vi "Create control.vi"() -> ()   [LabVIEW 2012]
uses:
  Typedefs/TypeDef_Action.ctl
  _Control Generator/BX.Orientation__LCR _Modified.ctl
  Controls/_ui_tools_font.ctl
  Control.lvclass
  <vilib>/Utility/miscctls.llb/LVPointTypeDef.ctl
  <vilib>/Palette API/Palette Menu/Public Type Define/Palette type.ctl
  <vilib>/Palette API/Palette Menu/Public Type Define/Item.ctl
  <userlib>/_OpenG.lib/array/array.llb/Conditional Auto-Indexing Tunnel (String)__ogtk.vi
  <userlib>/_OpenG.lib/file/file.llb/File Exists - Scalar__ogtk.vi
  <userlib>/_OpenG.lib/file/file.llb/Strip Path - Traditional__ogtk.vi
  <userlib>/_OpenG.lib/file/file.llb/Strip Path Extension - String__ogtk.vi
  <userlib>/_OpenG.lib/string/string.llb/To Proper Case (String)__ogtk.vi
  <vilib>/Utility/config.llb/Read Key (String).vi
  <vilib>/Utility/config.llb/Write Key (String).vi
  <vilib>/Utility/config.llb/Read Key (Boolean).vi
  <userlib>/_OpenG.lib/file/file.llb/Build Path - Traditional__ogtk.vi
  <vilib>/Utility/config.llb/NI_LVConfig.lvlib
  <vilib>/Palette API/Palette Menu/Palette Menu.lvlib
panel:
  in  "End program afterwards":bool
  in  "Save for version":u16(ring) items=["9.0", "8.6", "8.5", "8.2", "8.0"]
  in  "Save *.ctl to disk":bool
  in  "Zoom Min":bool
  in  "Zoom Max":bool
  in  "Scale Icon":dbl(slide)=1.0 min=0.5 max=2.0 scale=0.5..2.0 scale format="%.2g"
  in  "Text Color":u32(colorbox)
  in  "Palette":path=path "_LavaCR/CustomControls" caption="<user.lib>\\"
  in  "Front Panels":u16(ring)
  in  "Drop on Front Panel":bool
  in  "Font":T1={"Font Name:"="Tahoma", "Size"=13, "Strikeout?"=FALSE, "Italic?"=FALSE, "Underline?"=FALSE, "Outline?"=FALSE, "Shadow?"=FALSE, "Bold?"=TRUE}
  in  "Add a copy to UI Tools Palette":bool
  in  "Projects":u16(ring)
  in  "Add to Project":bool
  in  "Button Style":u16(ring) items=["GlassWeb", "Mac", "Mandelbrot", "OfficeXP", "Outlook", "Round", "System", "System_test", "Vista1", "Vista_medium", "Vista_small"]
  in  "Cancel":bool
  in  "Create":bool
  in  "Orientations":T2=14
  in  "Action":T3=4 items=["Switch when pressed", "Switch when released", "Switch until release", "Latch when pressed", "Latch when released", "Latch until released"]
  in  "Control Text":string
  in  "Icon source":path caption="Icon source (single PNG file or source directory for batch processing)"
  out "Controls preview":picture
  # "BATCH PROCESSING NOT IMPLEMENTED YET\nWITH THIS UTILITY VI."
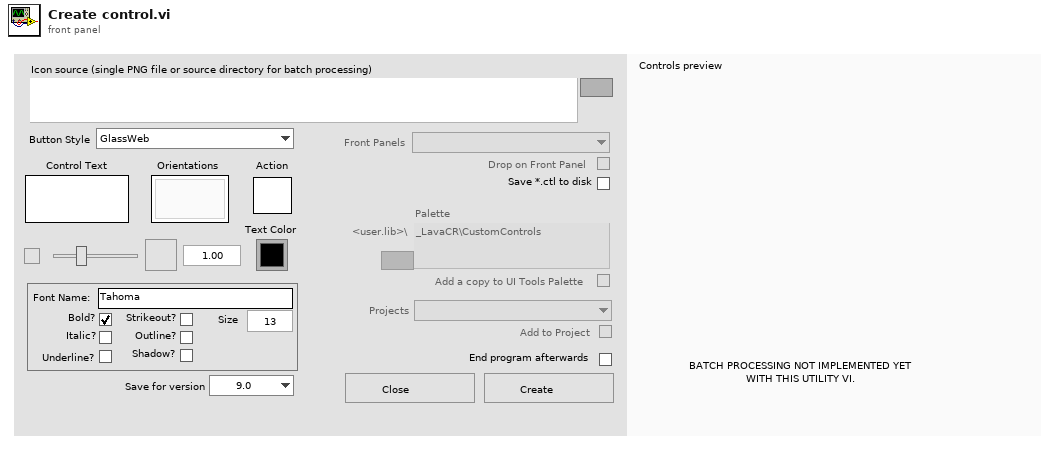
[diagram p1: front panel]
types:
  T1 = typedef "Control.lvclass/_ui_tools_font.ctl" = cluster{"Font Name:":string, "Size":i16, "Strikeout?":bool, "Italic?":bool, "Underline?":bool, "Outline?":bool, "Shadow?":bool, "Bold?":bool}
  T2 = typedef "BX.Orientation__LCR _Modified.ctl" = u8
  T3 = typedef "Control.lvclass/TypeDef_Action.ctl" = u16
  T4 = cluster{"Action":refnum<user-event>, "Orientations":refnum<user-event>, "Icon (*.png)":refnum<user-event>, "Font":refnum<user-event>, "Control Text":refnum<user-event>, "Style":refnum<user-event>, "Text Color":refnum<user-event>, "Scale Icon":refnum<user-event>}
  T5 = enum32{"invalid app kind", "Development System", "Run Time System", "Student Edition", "Embedded LabVIEW", "Evaluation", "Custom"}
  T6 = enum32{"Invalid", "Standard", "Closed", "Hidden", "Minimized", "Maximized"}
  T7 = enum32{"Bad", "Idle", "Run top level", "Running"}
  T8 = typedef "LVPointTypeDef.ctl" = cluster{"Horizontal":i16, "Vertical":i16}
  T9 = typedef "Palette Menu.lvlib/Item.ctl" = cluster{"item path":path, "library path (.lvlib)":path, "use default lvlib palette":bool, "short name":string, "place VI contents":bool, "hide synchronized item":bool, "reserve spot for synch item":bool, "configure when placing VI contents":bool}
  T10 = cluster{"Core":cluster{"Current VI Reference":refnum<vi>, "Close Panel on Exit?":bool, "NI.LV.Dialog namespace":bool, "Menu Launch:App":refnum<vi>, "Local App":refnum<vi>}, "Control":refnum<class "Control.lvclass">, "Errors":cluster{"code":i32, "Short":string, "Long":string, "Critical":bool}[], "user events":cluster{"Action":refnum<user-event>, "Orientations":refnum<user-event>, "Icon (*.png)":refnum<user-event>, "Font":refnum<user-event>, "Control Text":refnum<user-event>, "Style":refnum<user-event>, "Text Color":refnum<user-event>, "Scale Icon":refnum<user-event>}, "last state":cluster{"Action":T3, "Orientations":T2, "Icon png":path, "Control Text":string, "Style":u16, "Text Color":u32, "Scale":dbl, "Close afterwards":bool}, "config":cluster{"fade":u32, "droplabel":bool}, "file in tmp dir":path, "Source":cluster{"Icon source":path}}
  T11 = cluster{"code":i32, "Short":string, "Long":string, "Critical":bool}[]
  T12 = cluster{"Action":T3, "Orientations":T2, "Icon png":path, "Control Text":string, "Style":u16, "Text Color":u32, "Scale":dbl, "Close afterwards":bool}
  T13 = cluster{"Current VI Reference":refnum<vi>, "Close Panel on Exit?":bool, "NI.LV.Dialog namespace":bool, "Menu Launch:App":refnum<vi>, "Local App":refnum<vi>}
  T14 = typedef "NI_LVConfig.lvlib/Config Data RefNum.ctl" = refnum<k1>
  T15 = typedef "imagedata.ctl" = cluster{"image type":i32, "image depth":i32, "image":u8[], "mask":u8[], "colors":u32[], "Rectangle":cluster{"left":i16, "top":i16, "right":i16, "bottom":i16}}
  T16 = cluster{"left":i16, "top":i16, "right":i16, "bottom":i16}
  T17 = cluster{"code":i32, "Short":string, "Long":string, "Critical":bool}
  T18 = typedef "Palette Menu.lvlib/Palette type.ctl" = i32
  T19 = typedef "Palette Menu.lvlib/Palette Data.ctl" = cluster{"display name":string, "view format":T20, "palette width":i16, "items":T21, "256 color icon":picture, "B&W color icon":picture, "help information":T22, "palette description":string, "synchronize information":T23}
  T20 = typedef "Palette Menu.lvlib/View Format.ctl" = u16
  T21 = typedef "Palette Menu.lvlib/Items.ctl" = T9[]
  T22 = typedef "Palette Menu.lvlib/Help Info.ctl" = cluster{"help tag":string, "help file path ":path}
  T23 = typedef "Palette Menu.lvlib/Synchronize Info.ctl" = cluster{"synchronize with directory":bool, "synchronize directory path":path}
  T24 = typedef "Control.lvclass/BX.Orientation__LCR _Modified.ctl" = u8
  T25 = typedef "Control.lvclass/TypeDef_Styles.ctl" = u16
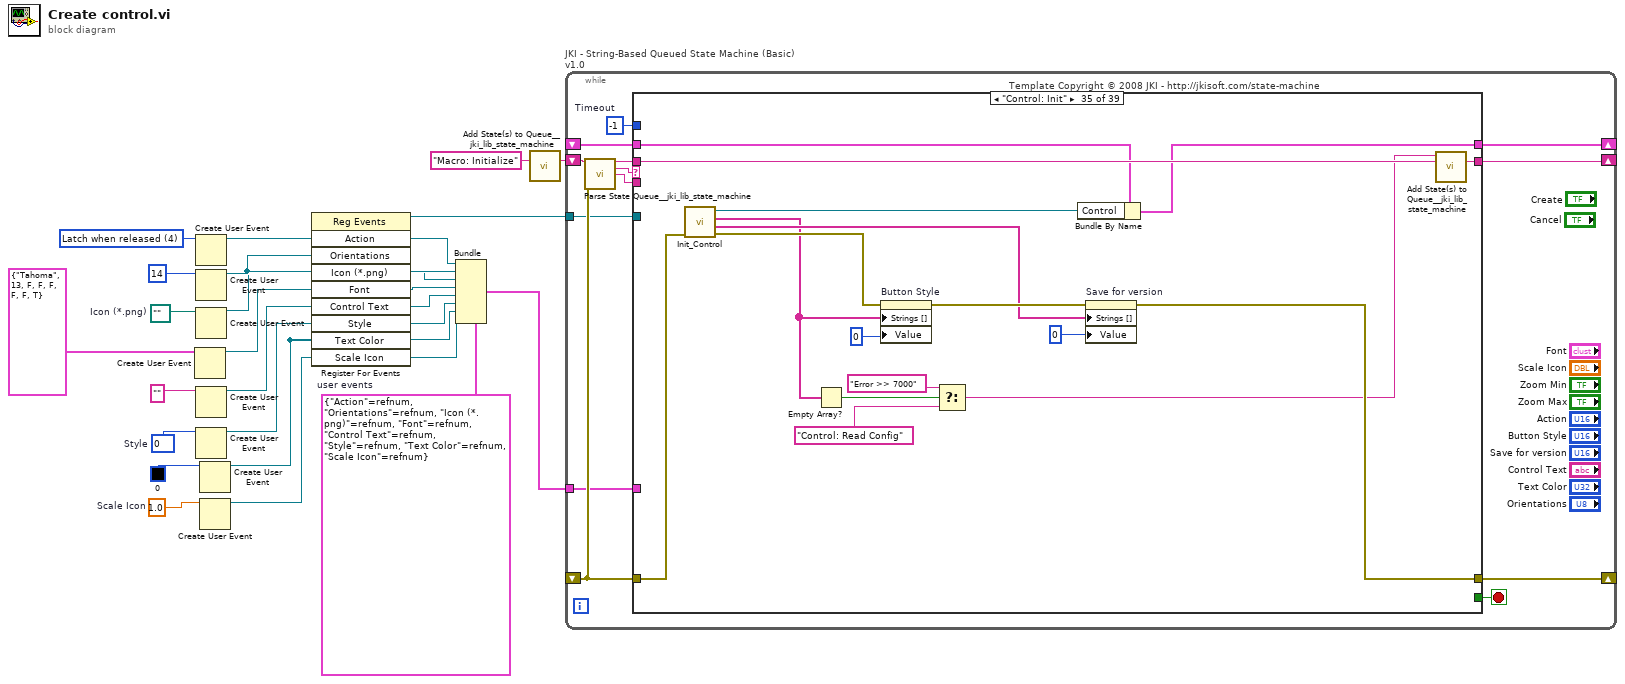
[diagram p0: block diagram]
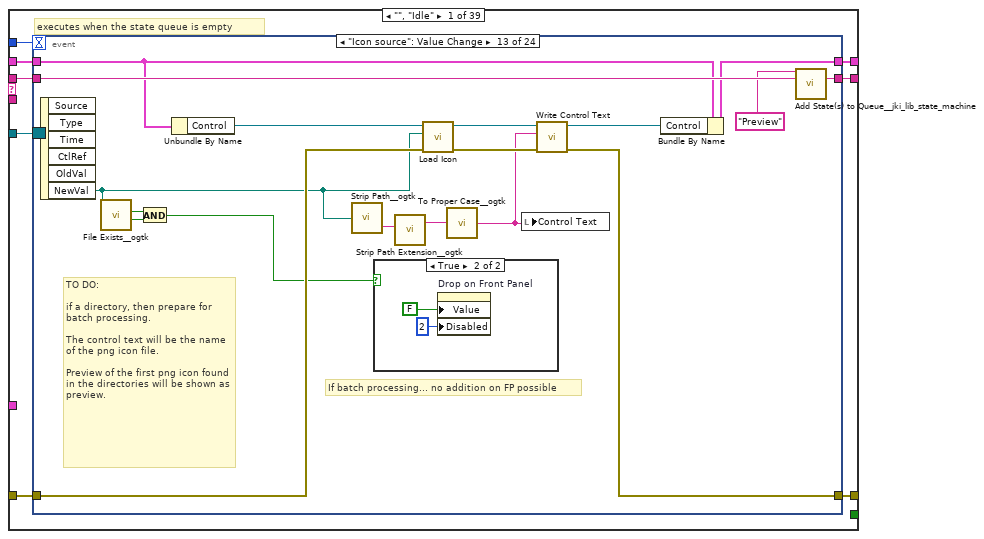
[diagram p2: hidden frame]
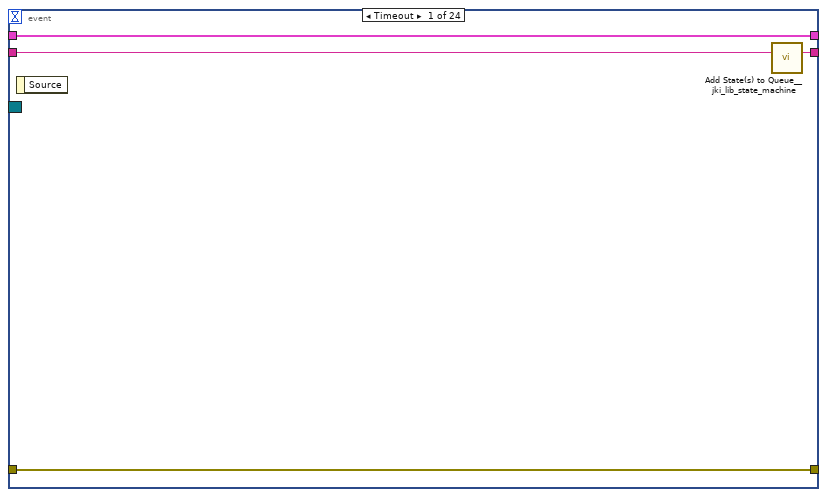
[diagram p3: hidden frame]
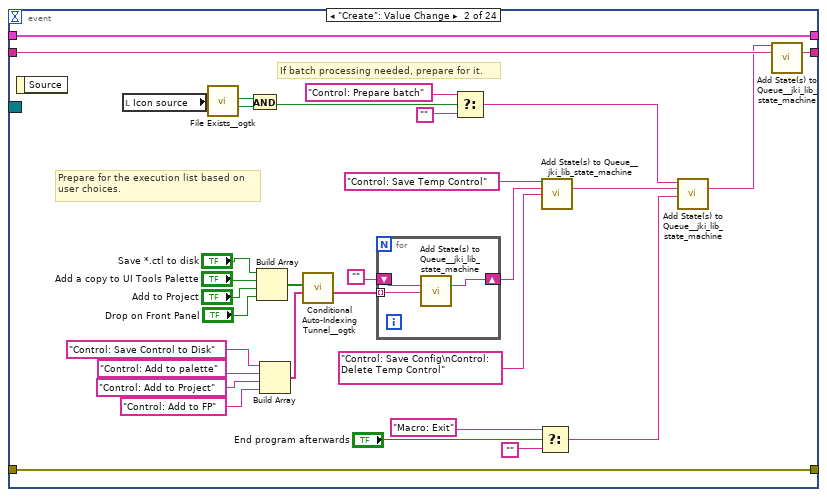
[diagram p4: hidden frame]
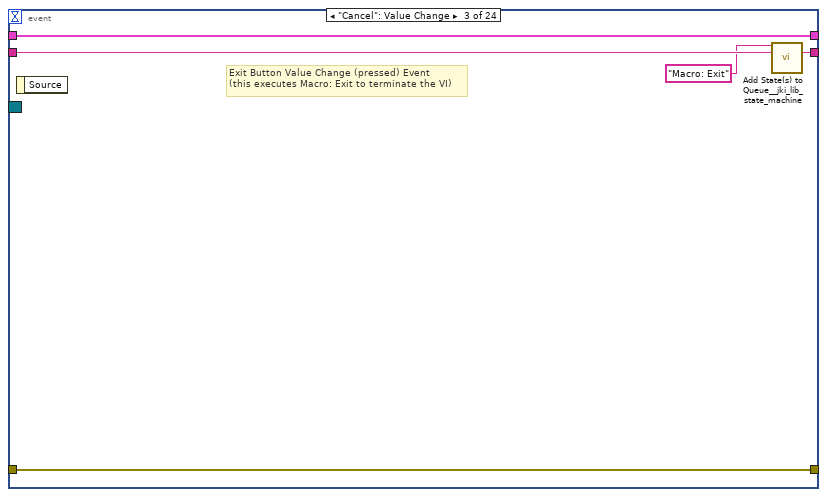
[diagram p5: hidden frame]
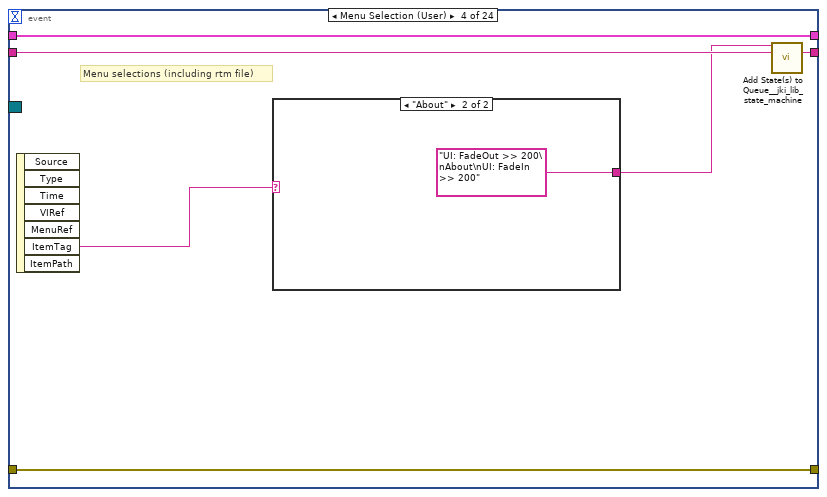
[diagram p6: hidden frame]
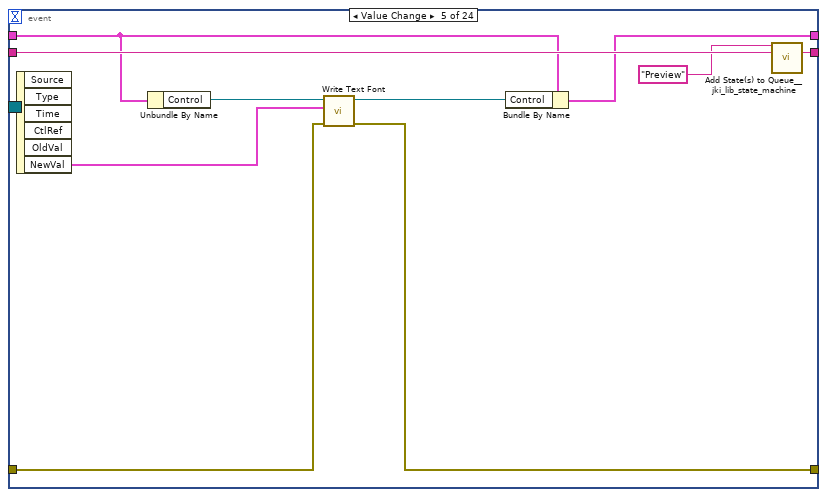
[diagram p8: hidden frame]
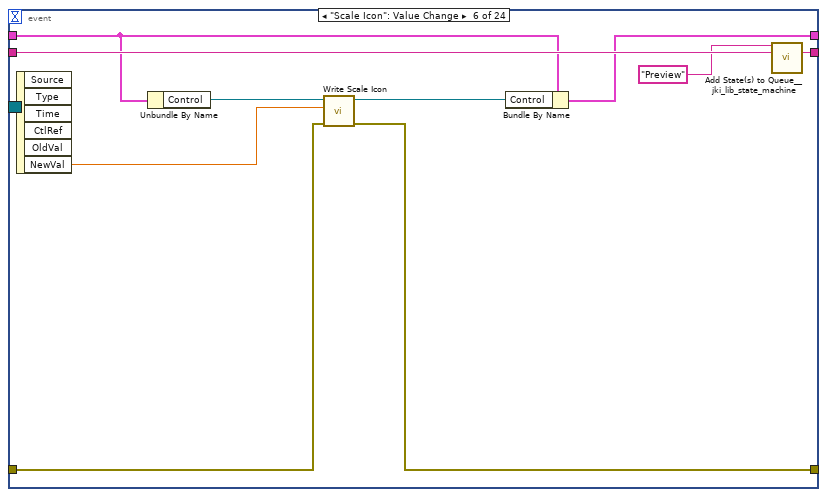
[diagram p9: hidden frame]
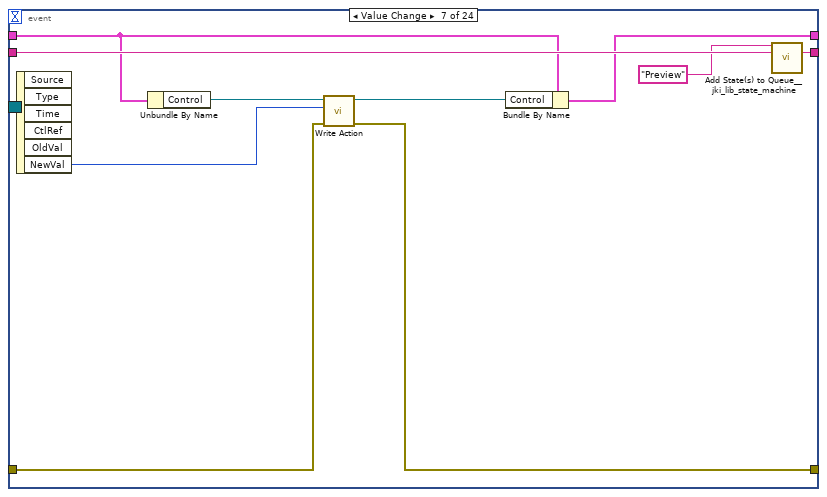
[diagram p10: hidden frame]
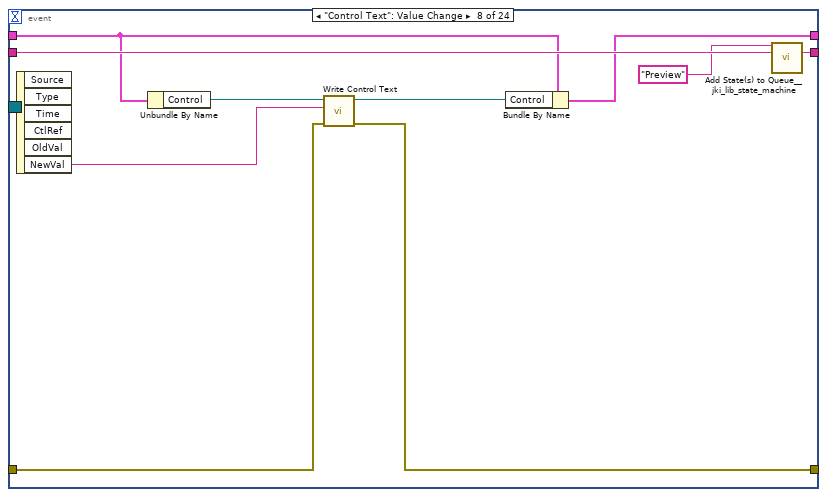
[diagram p11: hidden frame]
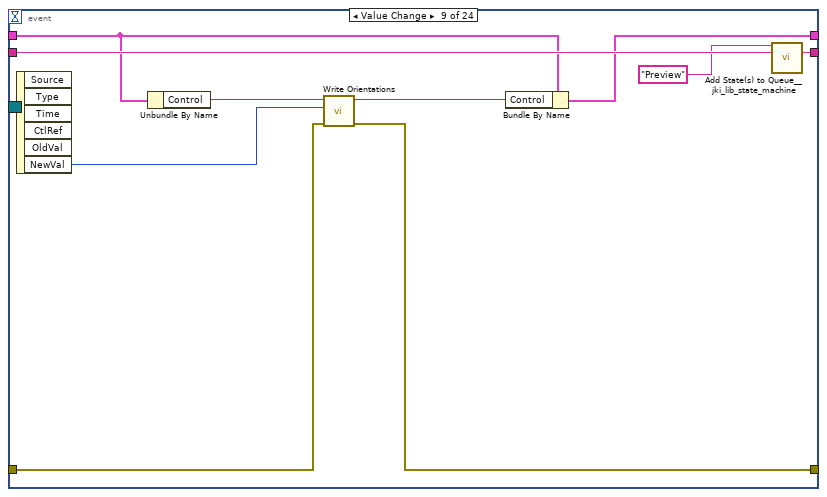
[diagram p12: hidden frame]
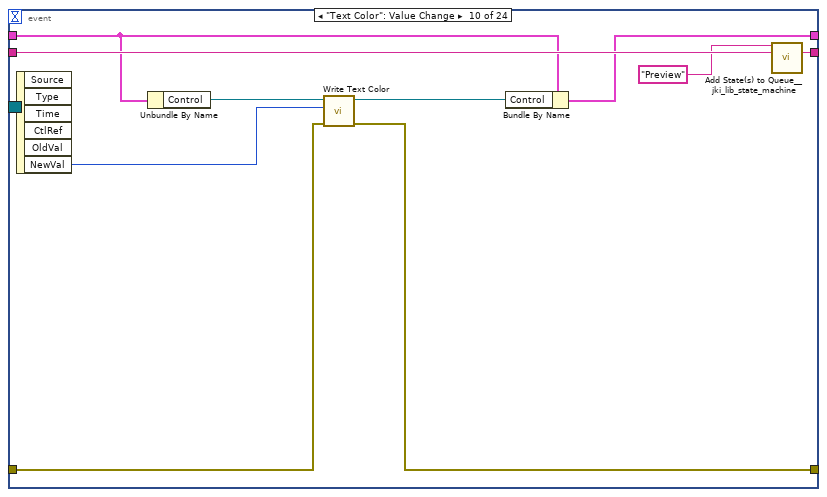
[diagram p13: hidden frame]
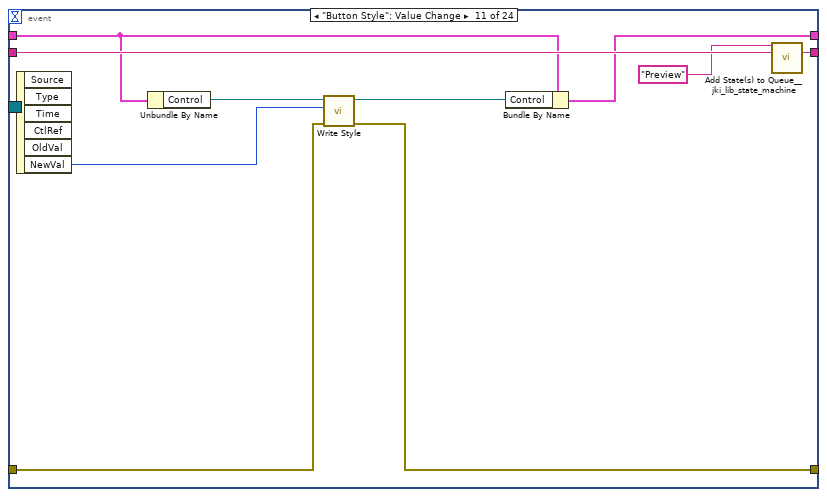
[diagram p14: hidden frame]
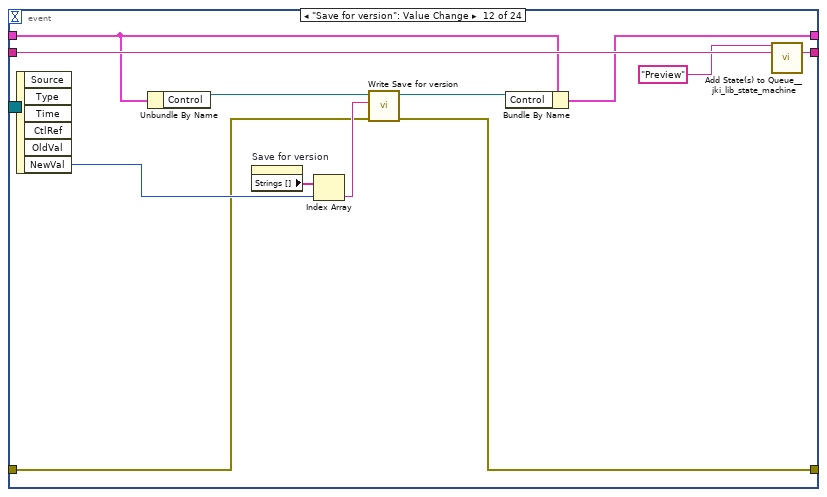
[diagram p15: hidden frame]
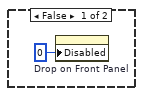
[diagram p16: hidden frame]
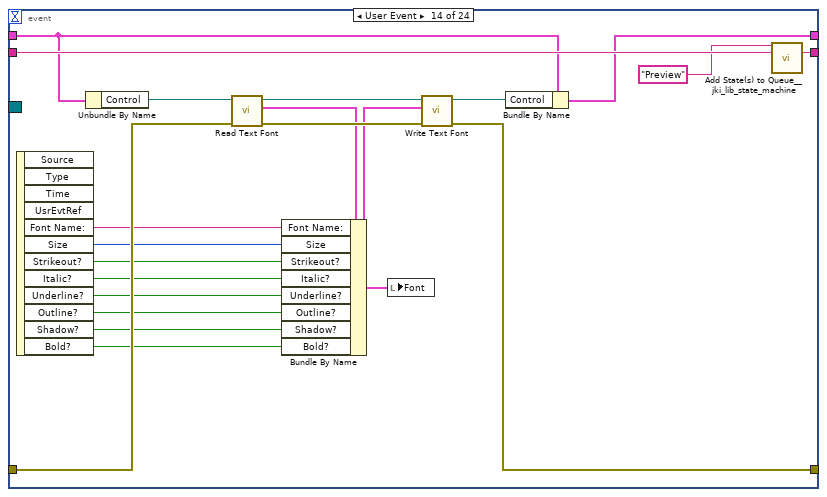
[diagram p17: hidden frame]
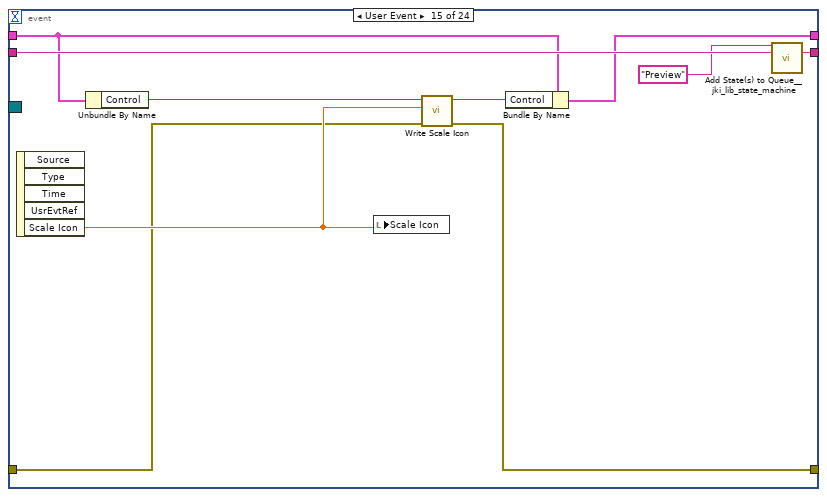
[diagram p18: hidden frame]
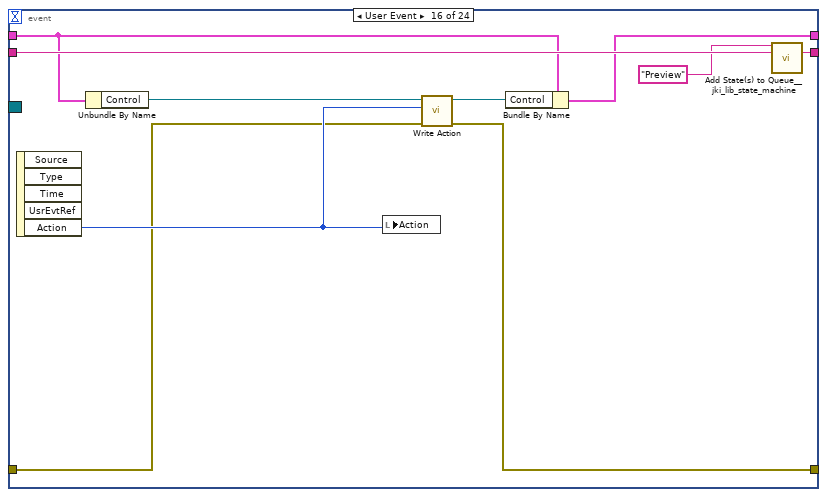
[diagram p19: hidden frame]
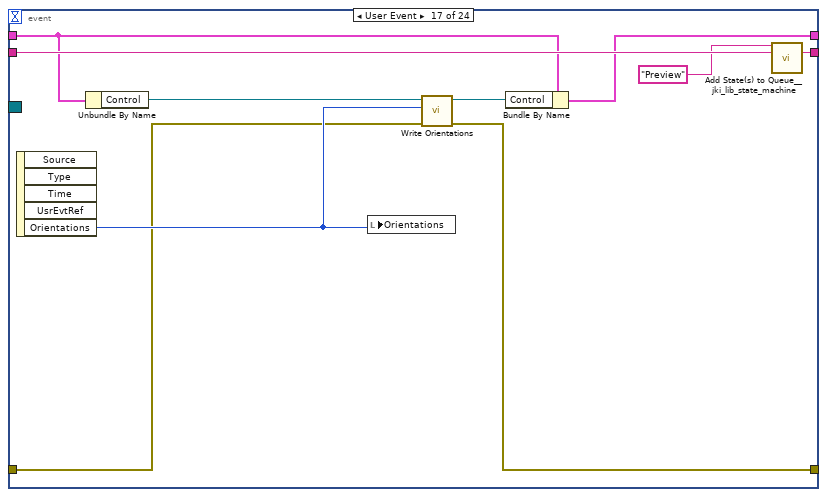
[diagram p20: hidden frame]
diagram:
  w2 = T4 {"Action"=refnum, "Orientations"=refnum, "Icon (*.png)"=refnum, "Font"=refnum, "Control Text"=refnum, "Style"=refnum, "Text Color"=refnum, "Scale Icon"=refnum}  # user events
  w7 = 1.0  # Scale Icon
  w11 = u16 0 items=[""]  # Style
  w17 = path ""  # Icon (*.png)
  w21 = T3 4 items=["Switch when pressed", "Switch when released", "Switch until release", "Latch when pressed", "Latch when released", "Latch until released"] ("Action")
  n1 = Create User Event(user event datatype=T1 {"Font Name:"="Tahoma", "Size"=13, "Strikeout?"=FALSE, "Italic?"=FALSE, "Underline?"=FALSE, "Outline?"=FALSE, "Shadow?"=FALSE, "Bold?"=TRUE} ("Font")) -> (user event=w14:refnum<user-event>)  [unwired: 1 in, 1 out]
  n2 = Create User Event(user event datatype=w21) -> (user event=w20:refnum<user-event>)  [unwired: 1 in, 1 out]
  n3 = Create User Event(user event datatype=T2 14 ("Orientations")) -> (user event=w19:refnum<user-event>)  [unwired: 1 in, 1 out]
  n4 = Create User Event(user event datatype=w17) -> (user event=w16:refnum<user-event>)  [unwired: 1 in, 1 out]
  n5 = Create User Event(user event datatype="" ("Control Text")) -> (user event=w12:refnum<user-event>)  [unwired: 1 in, 1 out]
  n6 = Create User Event(user event datatype=w11) -> (user event=w10:refnum<user-event>)  [unwired: 1 in, 1 out]
  n7 = Create User Event(user event datatype=u32 0 ("Text Color")) -> (user event=w8:refnum<user-event>)  [unwired: 1 in, 1 out]
  n8 = Create User Event(user event datatype=w7) -> (user event=w6:refnum<user-event>)  [unwired: 1 in, 1 out]
  n9 = register-events(w20, w19, w16, w14, w12, w10, w8, w6) -> (reference out=w1:refnum<event-registration>)  [unwired: 2 in, 1 out]
  n10 = Bundle(cluster=w2, "Action"=w20, "Orientations"=w19, "Icon (*.png)"=w16, "Font"=w14, "Control Text"=w12, "Style"=w10, "Text Color"=w8, "Scale Icon"=w6) -> (w3:T4)
  n11 = call <vilib>:"Add State(s) to Queue__jki_lib_state_machine.vi"("State(s) in (\"\")"="Macro: Initialize") -> ("States Out"=w5:string)  [unwired: 14 in]
  n12 = while "JKI - String-Based Queued State Machine (Basic) v1.0" {
    shift-right: [w27] -> _
    shift-left: _ -> [w26]
    shift-right: [w30] -> _
    shift-left: _ -> [w24]
    shift-right: [w29] -> _
    shift-left: w5 -> [w31]
    tunnel: w3 -> [w23]
    tunnel: w1 -> [w22]
    stop <- w28 stop-if-true
    w25 = -1  # Timeout
    # "Template Copyright © 2008 JKI - http://jkisoft.com/state-machine"
    n13 = call <vilib>:"Parse State Queue__jki_lib_state_machine.vi"("State Queue"=w31, "Error In (no error)"=w24) -> ("Remaining States"=w33:string, "Current State"=w34:string, "Arguments"=w32:string)  [unwired: 11 in]
    n14 = case shown="\"Control: Init\"" w34 {
      selector: w34 -> [_ _ w326 _ _ _ _ _ _ _ _ _ _ _ _ _ _ _ _ _ _ _ _ _ _ _ _ _ _ _ _ _ _ _ _ _ _ _ _]
      tunnel: w33 -> [w42 w325 w330 w340 w358 w368 w393 w403 w407 w419 w441 w454 w465 w492 w506 w513 w520 w526 w537 w576 w597 w620 w625 w636 w640 w661 w690 w730 w738 w761 w809 w841 w884 w904 w921 w933 w985 w1022 w1054]
      tunnel: w32 -> [_ _ _ _ _ _ w391 _ _ _ _ _ _ _ w502 _ _ w521 w531 _ _ _ _ _ _ _ _ _ _ _ _ _ _ _ _ _ _ _ _]
      tunnel: w26 -> [w40 w322 w328 w337 w349 w365 w390 w401 w404 _ w437 w451 w457 w477 w504 w511 w518 w524 w533 w561 w584 w617 w622 w628 w637 w645 w675 w727 w735 w759 w790 w839 w843 w901 w919 w934 w983 w1029 w1041]
      tunnel: [w39 w323 w332 w338 w355 errorcluster {"status"=FALSE, "code"=0, "source"=""} ("error out") w387 w400 w405 w416 w426 w452 w455 w480 w497 w508 w515 w522 w534 w574 w595 w618 w623 w626 w638 w659 w688 w728 w736 w742 w798 w831 w856 w902 w911 w939 w987 w1009 w1035] -> w30
      tunnel: w24 -> [w38 w323 w331 w338 w355 w360 _ w400 w405 w416 w438 w452 w455 w481 w498 w509 w516 w523 w535 w574 w595 w618 w623 w626 w638 w659 w688 w728 w736 w741 w797 w832 w861 w902 w912 w940 w988 w1008 w1036]
      tunnel: [w41 w324 w329 w339 w357 w367 w392 w402 w406 w418 w440 w453 w464 w491 w505 w512 w519 w525 w536 w575 w596 w619 w624 w635 w639 w660 w689 w729 w737 w760 w808 w840 w883 w903 w920 w937 w986 w1020 w1053] -> w29
      tunnel: [_ _ _ _ _ _ _ TRUE _ _ _ _ _ _ _ _ _ _ _ _ _ _ _ _ _ _ _ _ _ _ _ _ _ _ _ _ _ _ _] -> w28
      tunnel: [w37 w322 w328 w337 w356 w365 w390 w401 w404 w417 w437 w451 w457 w476 w504 w511 w518 w524 w533 w561 w584 w617 w622 w628 w637 w644 w674 w726 w734 w758 w807 w838 w882 w900 w918 w930 w984 w1029 w1040] -> w27
      tunnel: w25 -> [w36 _ _ _ _ _ _ _ _ _ _ _ _ _ _ _ _ _ _ _ _ _ _ _ _ _ _ _ _ _ _ _ _ _ _ _ _ _ _]
      tunnel: w23 -> [_ _ _ _ _ _ _ _ _ w412 _ _ _ _ _ _ _ _ _ _ _ _ _ _ _ _ _ _ _ _ _ _ _ _ _ _ _ _ _]
      tunnel: w22 -> [w35 _ _ _ _ _ _ _ _ _ w436 _ _ _ _ _ _ _ _ _ _ _ _ _ _ _ _ _ _ _ _ _ _ _ _ _ _ _ _]
      frame "", "Idle" {
        # "executes when the state queue is empty"
        n15 = event shown="[12] \"Icon source\": Value Change" {
          selector: w35 -> [_ _ _ _ _ _ _ _ _ _ _ _ _ _ _ _ _ _ _ _ _ _ _ _]
          dyn-events: _ -> [_ _ _ _ _ _ _ _ _ _ _ _ _ _ _ _ _ _ _ _ _ _ _ _]
          timeout: w36 -> [_ _ _ _ _ _ _ _ _ _ _ _ _ _ _ _ _ _ _ _ _ _ _ _]
          tunnel: w42 -> [w46 w78 w86 w92 w103 w113 w123 w133 w143 w153 w163 w175 w193 w217 w227 w237 w247 w257 w267 w277 w295 w305 w315 w321]
          tunnel: [w45 w77 w85 w91 w102 w112 w122 w132 w142 w152 w162 w174 w192 w216 w226 w236 w246 w256 w266 w276 w294 w304 w314 w320] -> w41
          tunnel: w40 -> [w43 w75 w83 w89 w100 w110 w120 w130 w140 w150 w160 w172 w190 w214 w224 w234 w244 w254 w264 w274 w292 w302 w312 w318]
          tunnel: [w44 w76 w84 w90 w94 w104 w114 w124 w134 w144 w154 w164 w182 w211 w221 w231 w241 w251 w261 w271 w282 w296 w306 w319] -> w39
          tunnel: w38 -> [w44 w76 w84 w90 w95 w105 w115 w125 w135 w145 w155 w165 w181 w207 w218 w228 w238 w248 w259 w269 w285 w297 w307 w319]
          tunnel: [w43 w75 w83 w89 w99 w109 w119 w129 w139 w149 w159 w171 w189 w213 w223 w233 w243 w253 w263 w273 w291 w301 w311 w318] -> w37
          event Timeout {
            n16 = event-data() -> ()  [unwired: 2 out]
            n17 = call <vilib>:"Add State(s) to Queue__jki_lib_state_machine.vi"("State(s) in (\"\")"=w46) -> ("States Out"=w45:string)  [unwired: 14 in]
          }
          event "Create": Value Change {
            # "If batch processing needed, prepare for it."
            # "Prepare for the execution list based on\nuser choices."
            n18 = event-data() -> ()  [unwired: 2 out]
            n19 = local read "Icon source"() -> (w59:path)
            n20 = call-poly <userlib>:"File Exists__ogtk.vi"("file path"=w59) -> ("is directory"=w58:bool, "exists"=w57:bool)  [unwired: 6 in]
            n21 = And(x=w58, y=w57) -> (x .and. y?=w53:bool)
            n22 = Build Array("Save *.ctl to disk", "Add a copy to UI Tools Palette", "Add to Project", "Drop on Front Panel") -> (w64:bool[])
            n23 = Build Array("Control: Save Control to Disk", "Control: Add to palette", "Control: Add to Project", "Control: Add to FP") -> (w63:string[])
            n24 = call-poly <userlib>:"Conditional Auto-Indexing Tunnel__ogtk.vi"("Array in"=w63, "Elements to keep"=w64) -> ("Filtered Array out"=w62:string[])  [unwired: 5 out]
            n25 = for {
              tunnel: w62 -> [w81] mode=indexing
              shift-right: [w79] -> w60
              shift-left: "" -> [w80]
              n26 = call <vilib>:"Add State(s) to Queue__jki_lib_state_machine.vi"("State(s) in (\"\")"=w80, "State(s) at Back (\"\")"=w81) -> ("States Out"=w79:string)  [unwired: 13 in]
            }
            n27 = Select(t="Control: Prepare batch", s=w53, f="") -> (s? t:f=w51:string)
            n28 = Select(t="Macro: Exit", s="End program afterwards", f="") -> (s? t:f=w47:string)
            n29 = call <vilib>:"Add State(s) to Queue__jki_lib_state_machine.vi"("State(s) in Front (\"\")"="Control: Save Temp Control", "State(s) in (\"\")"=w60, "State(s) at Back (\"\")"="Control: Save Config\nControl: Delete Temp Control") -> ("States Out"=w56:string)  [unwired: 12 in]
            n30 = call <vilib>:"Add State(s) to Queue__jki_lib_state_machine.vi"("State(s) in Front (\"\")"=w51, "State(s) in (\"\")"=w56, "State(s) at Back (\"\")"=w47) -> ("States Out"=w55:string)  [unwired: 12 in]
            n31 = call <vilib>:"Add State(s) to Queue__jki_lib_state_machine.vi"("State(s) in Front (\"\")"=w55, "State(s) in (\"\")"=w78) -> ("States Out"=w77:string)  [unwired: 13 in]
          }
          event "Cancel": Value Change {
            # "Exit Button Value Change (pressed) Event\n(this executes Macro: Exit to terminate the VI)"
            n32 = event-data() -> ()  [unwired: 2 out]
            n33 = call <vilib>:"Add State(s) to Queue__jki_lib_state_machine.vi"("State(s) in Front (\"\")"="Macro: Exit", "State(s) in (\"\")"=w86) -> ("States Out"=w85:string)  [unwired: 13 in]
          }
          event Menu Selection (User) {
            # "Menu selections (including rtm file)"
            n34 = event-data() -> ("ItemTag"=w87:string)  [unwired: 7 out]
            n35 = case shown="\"About\"" w87 {
              tunnel: [_ "UI: FadeOut >> 200\nAbout\nUI: FadeIn >> 200"] -> w88
              frame Default {
              }
              frame "About" {
              }
            }
            n36 = call <vilib>:"Add State(s) to Queue__jki_lib_state_machine.vi"("State(s) in Front (\"\")"=w88, "State(s) in (\"\")"=w92) -> ("States Out"=w91:string)  [unwired: 13 in]
          }
          event Value Change {
            n37 = event-data() -> ("NewVal"=w96:T1)  [unwired: 6 out]
            n38 = Unbundle By Name(w100) -> ("Control"=w98:refnum<class "Control.lvclass">)
            n39 = call-dynamic "Write Text Font.vi"("error in (no error)"=w95, "Font"=w96, "Control in"=w98) -> ("error out"=w94:errorcluster, "Control out"=w97:refnum<class "Control.lvclass">)  [unwired: 7 out]
            n40 = Bundle By Name(cluster=w100, "Control"=w97) -> (w99:T10)
            n41 = call <vilib>:"Add State(s) to Queue__jki_lib_state_machine.vi"("State(s) in Front (\"\")"="Preview", "State(s) in (\"\")"=w103) -> ("States Out"=w102:string)  [unwired: 13 in]
          }
          event "Scale Icon": Value Change {
            n42 = event-data() -> ("NewVal"=w106:dbl)  [unwired: 6 out]
            n43 = Unbundle By Name(w110) -> ("Control"=w108:refnum<class "Control.lvclass">)
            n44 = call-dynamic "Write Scale Icon.vi"("error in (no error)"=w105, "Scale Icon"=w106, "Control in"=w108) -> ("error out"=w104:errorcluster, "Control out"=w107:refnum<class "Control.lvclass">)  [unwired: 7 out]
            n45 = Bundle By Name(cluster=w110, "Control"=w107) -> (w109:T10)
            n46 = call <vilib>:"Add State(s) to Queue__jki_lib_state_machine.vi"("State(s) in Front (\"\")"="Preview", "State(s) in (\"\")"=w113) -> ("States Out"=w112:string)  [unwired: 13 in]
          }
          event Value Change {
            n47 = event-data() -> ("NewVal"=w116:T3)  [unwired: 6 out]
            n48 = Unbundle By Name(w120) -> ("Control"=w118:refnum<class "Control.lvclass">)
            n49 = call-dynamic "Write Action.vi"("error in (no error)"=w115, "Action"=w116, "Control in"=w118) -> ("error out"=w114:errorcluster, "Control out"=w117:refnum<class "Control.lvclass">)  [unwired: 7 out]
            n50 = Bundle By Name(cluster=w120, "Control"=w117) -> (w119:T10)
            n51 = call <vilib>:"Add State(s) to Queue__jki_lib_state_machine.vi"("State(s) in Front (\"\")"="Preview", "State(s) in (\"\")"=w123) -> ("States Out"=w122:string)  [unwired: 13 in]
          }
          event "Control Text": Value Change {
            n52 = event-data() -> ("NewVal"=w126:string)  [unwired: 6 out]
            n53 = Unbundle By Name(w130) -> ("Control"=w128:refnum<class "Control.lvclass">)
            n54 = call-dynamic "Write Control Text.vi"("error in (no error)"=w125, "Control Text"=w126, "Control in"=w128) -> ("error out"=w124:errorcluster, "Control out"=w127:refnum<class "Control.lvclass">)  [unwired: 7 out]
            n55 = Bundle By Name(cluster=w130, "Control"=w127) -> (w129:T10)
            n56 = call <vilib>:"Add State(s) to Queue__jki_lib_state_machine.vi"("State(s) in Front (\"\")"="Preview", "State(s) in (\"\")"=w133) -> ("States Out"=w132:string)  [unwired: 13 in]
          }
          event Value Change {
            n57 = event-data() -> ("NewVal"=w136:T2)  [unwired: 6 out]
            n58 = Unbundle By Name(w140) -> ("Control"=w138:refnum<class "Control.lvclass">)
            n59 = call-dynamic "Write Orientations.vi"("error in (no error)"=w135, "Orientations"=w136, "Control in"=w138) -> ("error out"=w134:errorcluster, "Control out"=w137:refnum<class "Control.lvclass">)  [unwired: 7 out]
            n60 = Bundle By Name(cluster=w140, "Control"=w137) -> (w139:T10)
            n61 = call <vilib>:"Add State(s) to Queue__jki_lib_state_machine.vi"("State(s) in Front (\"\")"="Preview", "State(s) in (\"\")"=w143) -> ("States Out"=w142:string)  [unwired: 13 in]
          }
          event "Text Color": Value Change {
            n62 = event-data() -> ("NewVal"=w146:u32)  [unwired: 6 out]
            n63 = Unbundle By Name(w150) -> ("Control"=w148:refnum<class "Control.lvclass">)
            n64 = call-dynamic "Write Text Color.vi"("error in (no error)"=w145, "Text Color"=w146, "Control.lvclass in"=w148) -> ("error out"=w144:errorcluster, "Control.lvclass out"=w147:refnum<class "Control.lvclass">)  [unwired: 7 out]
            n65 = Bundle By Name(cluster=w150, "Control"=w147) -> (w149:T10)
            n66 = call <vilib>:"Add State(s) to Queue__jki_lib_state_machine.vi"("State(s) in Front (\"\")"="Preview", "State(s) in (\"\")"=w153) -> ("States Out"=w152:string)  [unwired: 13 in]
          }
          event "Button Style": Value Change {
            n67 = event-data() -> ("NewVal"=w156:u16)  [unwired: 6 out]
            n68 = Unbundle By Name(w160) -> ("Control"=w158:refnum<class "Control.lvclass">)
            n69 = call-dynamic "Write Style.vi"("error in (no error)"=w155, "Style index (-1)"=w156, "Control in"=w158) -> ("error out"=w154:errorcluster, "Control out"=w157:refnum<class "Control.lvclass">)  [unwired: 1 in, 6 out]
            n70 = Bundle By Name(cluster=w160, "Control"=w157) -> (w159:T10)
            n71 = call <vilib>:"Add State(s) to Queue__jki_lib_state_machine.vi"("State(s) in Front (\"\")"="Preview", "State(s) in (\"\")"=w163) -> ("States Out"=w162:string)  [unwired: 13 in]
          }
          event "Save for version": Value Change {
            n72 = event-data() -> ("NewVal"=w168:u16)  [unwired: 6 out]
            n73 = Unbundle By Name(w172) -> ("Control"=w167:refnum<class "Control.lvclass">)
            n74 = property on="Save for version" class="Ring (strict)"() -> ("Strings []"=w169:string[])  [unwired: 2 in, 2 out]
            n75 = Index Array(array=w169, index=w168) -> (element=w170:string)
            n76 = call-dynamic "Write Save for version.vi"("error in (no error)"=w165, "Save for version"=w170, "Control.lvclass in"=w167) -> ("error out"=w164:errorcluster, "Control.lvclass out"=w166:refnum<class "Control.lvclass">)  [unwired: 7 out]
            n77 = Bundle By Name(cluster=w172, "Control"=w166) -> (w171:T10)
            n78 = call <vilib>:"Add State(s) to Queue__jki_lib_state_machine.vi"("State(s) in Front (\"\")"="Preview", "State(s) in (\"\")"=w175) -> ("States Out"=w174:string)  [unwired: 13 in]
          }
          event "Icon source": Value Change {
            # "If batch processing... no addition on FP possible"
            # "TO DO: \n\nif a directory, then prepare for batch processing.\n\nThe control text will be the name of the png icon file.\n\nPreview of the first png icon found in the directories will be shown as preview."
            n79 = event-data() -> ("NewVal"=w179:path)  [unwired: 6 out]
            n80 = call-poly <userlib>:"File Exists__ogtk.vi"("file path"=w179) -> ("is directory"=w178:bool, "exists"=w177:bool)  [unwired: 6 in]
            n81 = And(x=w178, y=w177) -> (x .and. y?=w176:bool)
            n82 = Unbundle By Name(w190) -> ("Control"=w180:refnum<class "Control.lvclass">)
            n83 = call-poly <userlib>:"Strip Path__ogtk.vi"("path"=w179) -> ("name"=w188:string)  [unwired: 1 out]
            n84 = case shown="True" w176 {
              frame False {
                n85 = property on="Drop on Front Panel" class="Bool (strict)"("Disabled"=u8 0) -> ()  [unwired: 2 in, 2 out]
              }
              frame True {
                n86 = property on="Drop on Front Panel" class="Bool (strict)"("Value"=FALSE ("Drop on Front Panel"), "Disabled"=u8 2) -> ()  [unwired: 2 in, 2 out]
              }
            }
            n87 = call-poly <userlib>:"Strip Path Extension__ogtk.vi"("path"=w188) -> ("root"=w187:string)  [unwired: 1 out]
            n88 = call-dynamic "Load Icon.vi"("error in (no error)"=w181, "Icon path False"=w179, "Control in"=w180) -> ("error out"=w185:errorcluster, "Control out"=w186:refnum<class "Control.lvclass">)  [unwired: 1 in, 6 out]
            n89 = call-poly <userlib>:"To Proper Case__ogtk.vi"("string"=w187) -> ("proper case string"=w184:string)  [unwired: 4 out]
            n90 = local write "Control Text"(w184) -> ()
            n91 = call-dynamic "Write Control Text.vi"("error in (no error)"=w185, "Control Text"=w184, "Control in"=w186) -> ("error out"=w182:errorcluster, "Control out"=w183:refnum<class "Control.lvclass">)  [unwired: 7 out]
            n92 = Bundle By Name(cluster=w190, "Control"=w183) -> (w189:T10)
            n93 = call <vilib>:"Add State(s) to Queue__jki_lib_state_machine.vi"("State(s) in Front (\"\")"="Preview", "State(s) in (\"\")"=w193) -> ("States Out"=w192:string)  [unwired: 13 in]
          }
          event User Event {
            n94 = event-data() -> ("Font Name:"=w205:string, "Size"=w204:i16, "Strikeout?"=w203:bool, "Italic?"=w202:bool, "Underline?"=w201:bool, "Outline?"=w200:bool, "Shadow?"=w199:bool, "Bold?"=w198:bool)  [unwired: 5 out]
            n95 = Unbundle By Name(w214) -> ("Control"=w209:refnum<class "Control.lvclass">)
            n96 = call-dynamic "Read Text Font.vi"("error in (no error)"=w207, "Control in"=w209) -> ("error out"=w208:errorcluster, "Font"=w206:T1, "Control out"=w210:refnum<class "Control.lvclass">)  [unwired: 7 out]
            n97 = Bundle By Name(cluster=w206, "Font Name:"=w205, "Size"=w204, "Strikeout?"=w203, "Italic?"=w202, "Underline?"=w201, "Outline?"=w200, "Shadow?"=w199, "Bold?"=w198) -> (w197:T1)
            n98 = local write "Font"(w197) -> ()
            n99 = call-dynamic "Write Text Font.vi"("error in (no error)"=w208, "Font"=w197, "Control in"=w210) -> ("error out"=w211:errorcluster, "Control out"=w212:refnum<class "Control.lvclass">)  [unwired: 7 out]
            n100 = Bundle By Name(cluster=w214, "Control"=w212) -> (w213:T10)
            n101 = call <vilib>:"Add State(s) to Queue__jki_lib_state_machine.vi"("State(s) in Front (\"\")"="Preview", "State(s) in (\"\")"=w217) -> ("States Out"=w216:string)  [unwired: 13 in]
          }
          event User Event {
            n102 = event-data() -> ("Scale Icon"=w220:dbl)  [unwired: 5 out]
            n103 = Unbundle By Name(w224) -> ("Control"=w219:refnum<class "Control.lvclass">)
            n104 = local write "Scale Icon"(w220) -> ()
            n105 = call-dynamic "Write Scale Icon.vi"("error in (no error)"=w218, "Scale Icon"=w220, "Control in"=w219) -> ("error out"=w221:errorcluster, "Control out"=w222:refnum<class "Control.lvclass">)  [unwired: 7 out]
            n106 = Bundle By Name(cluster=w224, "Control"=w222) -> (w223:T10)
            n107 = call <vilib>:"Add State(s) to Queue__jki_lib_state_machine.vi"("State(s) in Front (\"\")"="Preview", "State(s) in (\"\")"=w227) -> ("States Out"=w226:string)  [unwired: 13 in]
          }
          event User Event {
            n108 = event-data() -> ("Action"=w230:T3)  [unwired: 5 out]
            n109 = Unbundle By Name(w234) -> ("Control"=w229:refnum<class "Control.lvclass">)
            n110 = local write "Action"(w230) -> ()
            n111 = call-dynamic "Write Action.vi"("error in (no error)"=w228, "Action"=w230, "Control in"=w229) -> ("error out"=w231:errorcluster, "Control out"=w232:refnum<class "Control.lvclass">)  [unwired: 7 out]
            n112 = Bundle By Name(cluster=w234, "Control"=w232) -> (w233:T10)
            n113 = call <vilib>:"Add State(s) to Queue__jki_lib_state_machine.vi"("State(s) in Front (\"\")"="Preview", "State(s) in (\"\")"=w237) -> ("States Out"=w236:string)  [unwired: 13 in]
          }
          event User Event {
            n114 = event-data() -> ("Orientations"=w240:T2)  [unwired: 5 out]
            n115 = Unbundle By Name(w244) -> ("Control"=w239:refnum<class "Control.lvclass">)
            n116 = local write "Orientations"(w240) -> ()
            n117 = call-dynamic "Write Orientations.vi"("error in (no error)"=w238, "Orientations"=w240, "Control in"=w239) -> ("error out"=w241:errorcluster, "Control out"=w242:refnum<class "Control.lvclass">)  [unwired: 7 out]
            n118 = Bundle By Name(cluster=w244, "Control"=w242) -> (w243:T10)
            n119 = call <vilib>:"Add State(s) to Queue__jki_lib_state_machine.vi"("State(s) in Front (\"\")"="Preview", "State(s) in (\"\")"=w247) -> ("States Out"=w246:string)  [unwired: 13 in]
          }
          event User Event {
            n120 = event-data() -> ("Control Text"=w250:string)  [unwired: 5 out]
            n121 = Unbundle By Name(w254) -> ("Control"=w249:refnum<class "Control.lvclass">)
            n122 = local write "Control Text"(w250) -> ()
            n123 = call-dynamic "Write Control Text.vi"("error in (no error)"=w248, "Control Text"=w250, "Control in"=w249) -> ("error out"=w251:errorcluster, "Control out"=w252:refnum<class "Control.lvclass">)  [unwired: 7 out]
            n124 = Bundle By Name(cluster=w254, "Control"=w252) -> (w253:T10)
            n125 = call <vilib>:"Add State(s) to Queue__jki_lib_state_machine.vi"("State(s) in Front (\"\")"="Preview", "State(s) in (\"\")"=w257) -> ("States Out"=w256:string)  [unwired: 13 in]
          }
          event User Event {
            n126 = event-data() -> ("Style"=w258:u16)  [unwired: 5 out]
            n127 = Unbundle By Name(w264) -> ("Control"=w260:refnum<class "Control.lvclass">)
            n128 = local write "Button Style"(w258) -> ()
            n129 = call-dynamic "Write Style.vi"("error in (no error)"=w259, "Style index (-1)"=w258, "Control in"=w260) -> ("error out"=w261:errorcluster, "Control out"=w262:refnum<class "Control.lvclass">)  [unwired: 1 in, 6 out]
            n130 = Bundle By Name(cluster=w264, "Control"=w262) -> (w263:T10)
            n131 = call <vilib>:"Add State(s) to Queue__jki_lib_state_machine.vi"("State(s) in Front (\"\")"="Preview", "State(s) in (\"\")"=w267) -> ("States Out"=w266:string)  [unwired: 13 in]
          }
          event User Event {
            n132 = event-data() -> ("Text Color"=w268:u32)  [unwired: 5 out]
            n133 = Unbundle By Name(w274) -> ("Control"=w270:refnum<class "Control.lvclass">)
            n134 = local write "Text Color"(w268) -> ()
            n135 = call-dynamic "Write Text Color.vi"("error in (no error)"=w269, "Text Color"=w268, "Control.lvclass in"=w270) -> ("error out"=w271:errorcluster, "Control.lvclass out"=w272:refnum<class "Control.lvclass">)  [unwired: 7 out]
            n136 = Bundle By Name(cluster=w274, "Control"=w272) -> (w273:T10)
            n137 = call <vilib>:"Add State(s) to Queue__jki_lib_state_machine.vi"("State(s) in Front (\"\")"="Preview", "State(s) in (\"\")"=w277) -> ("States Out"=w276:string)  [unwired: 13 in]
          }
          event User Event {
            # "If the Control Text terminal is not empty, then do not override the user's input."
            n138 = event-data() -> ("Icon (*.png)"=w284:path)  [unwired: 5 out]
            n139 = Unbundle By Name(w292) -> ("Control"=w279:refnum<class "Control.lvclass">)
            n140 = local write "Icon source"(w284) -> ()
            n141 = call-poly <userlib>:"Strip Path__ogtk.vi"("path"=w284) -> ("name"=w287:string)  [unwired: 1 out]
            n142 = local read "Control Text"() -> (w289:string)
            n143 = call-poly <userlib>:"Strip Path Extension__ogtk.vi"("path"=w287) -> ("root"=w286:string)  [unwired: 1 out]
            n144 = call-dynamic "Load Icon.vi"("error in (no error)"=w285, "Icon path False"=w284, "Control in"=w279) -> ("error out"=w283:errorcluster, "Control out"=w280:refnum<class "Control.lvclass">)  [unwired: 1 in, 6 out]
            n145 = call-poly <userlib>:"To Proper Case__ogtk.vi"("string"=w286) -> ("proper case string"=w290:string)  [unwired: 4 out]
            n146 = Empty String/Path?(string/path=w289) -> (empty?=w288:bool)
            n147 = Select(t=w290, s=w288, f=w289) -> (s? t:f=w278:string)
            n148 = local write "Control Text"(w278) -> ()
            n149 = call-dynamic "Write Control Text.vi"("error in (no error)"=w283, "Control Text"=w278, "Control in"=w280) -> ("error out"=w282:errorcluster, "Control out"=w281:refnum<class "Control.lvclass">)  [unwired: 7 out]
            n150 = Bundle By Name(cluster=w292, "Control"=w281) -> (w291:T10)
            n151 = call <vilib>:"Add State(s) to Queue__jki_lib_state_machine.vi"("State(s) in Front (\"\")"="Preview", "State(s) in (\"\")"=w295) -> ("States Out"=w294:string)  [unwired: 13 in]
          }
          event "Zoom Min": Value Change {
            # "Zoomig is set from 0.5 to 2."
            n152 = event-data() -> ()  [unwired: 7 out]
            n153 = Unbundle By Name(w302) -> ("Control"=w299:refnum<class "Control.lvclass">, "user events.Scale Icon"=w298:refnum<user-event>)
            n154 = Generate User Event(user event=w298, event data cluster=0.5 ("event data"), error in=w297) -> (error out=w296:errorcluster)  [unwired: 1 out]
            n155 = Bundle By Name(cluster=w302, "Control"=w299) -> (w301:T10)
            n156 = call <vilib>:"Add State(s) to Queue__jki_lib_state_machine.vi"("State(s) in Front (\"\")"="Preview", "State(s) in (\"\")"=w305) -> ("States Out"=w304:string)  [unwired: 13 in]
          }
          event "Zoom Max": Value Change {
            # "Zoomig is set from 0.5 to 2."
            n157 = event-data() -> ()  [unwired: 7 out]
            n158 = Unbundle By Name(w312) -> ("Control"=w309:refnum<class "Control.lvclass">, "user events.Scale Icon"=w308:refnum<user-event>)
            n159 = Generate User Event(user event=w308, event data cluster=2.0 ("event data"), error in=w307) -> (error out=w306:errorcluster)  [unwired: 1 out]
            n160 = Bundle By Name(cluster=w312, "Control"=w309) -> (w311:T10)
            n161 = call <vilib>:"Add State(s) to Queue__jki_lib_state_machine.vi"("State(s) in Front (\"\")"="Preview", "State(s) in (\"\")"=w315) -> ("States Out"=w314:string)  [unwired: 13 in]
          }
          event Panel Close? {
            # "Discard the event because we'll close the front panel ourselves in Macro: Exit"
            # "Close Panel button (pressed) Event\n(this executes Macro: Exit to terminate the VI)"
            n162 = event-data() -> ()  [unwired: 2 out]
            n163 = event-data("Discard?"=TRUE) -> ()  [unwired: 1 in, 1 out]
            n164 = call <vilib>:"Add State(s) to Queue__jki_lib_state_machine.vi"("State(s) in Front (\"\")"="Macro: Exit", "State(s) in (\"\")"=w321) -> ("States Out"=w320:string)  [unwired: 13 in]
          }
        }
      }
      frame "---------- Core ----------" {
        # "Do not put any code in this frame.\n(it is a separator no-op)"
        n165 = call <vilib>:"Add State(s) to Queue__jki_lib_state_machine.vi"("State(s) in (\"\")"=w325) -> ("States Out"=w324:string)  [unwired: 14 in]
      }
      frame Default {
        w335 = 42 items=["No error", "Argument error", "Memory is full", "Out of zone", "End of file", "File already open", "Generic file I/O error", "File not found", "File permission error", "Disk is full", "Duplicate path", "Too many files open", "System feature not enabled", "Resource file not found", "Cannot add resource", "Resource not found", "Image not found", "Image memory error", "Pen does not exist", "Config type invalid", "Config token not found", "Config parse error", "Config memory error", "Bad external code format", "Bad external code offset", "External code not present", "Null window", "Destroy window error", "Null menu", "Print aborted", "Bad print record", "Print driver error", "Windows error during printing", "Memory error during printing", "Print dialog error", "Generic print error", "Invalid device refnum", "Device not found", "Device parameter error", "Device unit error", "Cannot open device", "Device call aborted", "Generic error", "Cancelled by user", "Object ID too low", "Object ID too high", "Object not in heap", "Unknown heap", "Unknown object (invalid DefProc)", "Unknown object (DefProc not in table)", "Message out of range", "Invalid (null) method", "Unknown message", "Manager call not supported", "Bad address", "Network operation in progress", "Network operation timed out", "Connection is busy", "Network attribute not supported", "Network error", "Address in use", "System out of memory", "Connection aborted", "Connection refused", "Not connected", "Already connected", "Connection closed", "Initialization error (interapplication manager)", "Bad occurrence", "Wait on unbound occurrence handler", "Occurrence queue overflow", "Datalog type conflict", "Unused", "Unrecognized type (interapplication manager)", "Memory corrupt", "Failed to make temporary DLL", "Old CIN version", "Drag socket not found", "Failed to load drop-object", "Failed to register OLE object", "Failed to release OLE object", "Format specifier type mismatch", "Unknown format specifier", "Too few format specifiers", "Too many format specifiers", "Scan failed", "Newer CIN version", "Error converting to variant", "Runtime menu error", "Password tampered", "Variant attribute not found", "Incompatible variant data type", "Event data is not available", "Event Store is not present", "Occurrence is not found", "Event Queue is not created", "Event info is not available", "Refnum passed is NULL", "Error retrieving Class GUID", "Error retrieving CoClass GUID", "Error retrieving TypeLib GUID.", "Bad built application magic bytes.", "Specific driver is different from the specific driver associated with the Logical Name.", "There is no session opened to the class driver.", "Max Error", "MAX - Error with config objects", "MAX - Error loading configuration", "MAX - Group not supported"]
        # "Current State"
        # "Do not delete, rename, or modify this frame.\n(this is used to capture unhandled states and typos)"
        # "Handle mistyped state name (developer tool)"
        n166 = Format Into String(format string="Software Exception: Unhandled State \"%s\"." ("message"), error in=w331, w326) -> (resulting string=w334:string, error out=w333:errorcluster)  [unwired: 1 in]
        n167 = call <vilib>:"Error Cluster From Error Code.vi"("show call chain? (False)"=TRUE, "error in (no error)"=w333, "error message (\"\")"=w334, "error code (0)"=w335) -> ("error out"=w332:errorcluster)  [unwired: 5 out]
        n168 = call <vilib>:"Add State(s) to Queue__jki_lib_state_machine.vi"("State(s) in (\"\")"=w330) -> ("States Out"=w329:string)  [unwired: 14 in]
      }
      frame "About" {
        n169 = call "About control creator.vi"() -> ()  [unwired: 12 out]
        n170 = call <vilib>:"Add State(s) to Queue__jki_lib_state_machine.vi"("State(s) in (\"\")"=w340) -> ("States Out"=w339:string)  [unwired: 14 in]
      }
      frame "Initialize Core Data" {
        # "If panel starts closed or is an EXE or is launched from Tools menu, then close it when we exit"
        # "Do not delete, rename, or modify this frame.\n(this is used to determine panel behavior on exit)"
        # "originally closed?"
        # "exe?"
        n171 = property class="Application"() -> (error out=w347:errorcluster, "App.MenuLaunchApp"=w345:refnum<vi>)  [unwired: 2 in, 1 out]
        n172 = property class="VI"() -> ("Front Panel.Open"=w354:bool)  [unwired: 2 in, 2 out]
        n173 = property class="App"() -> (reference out=w343:refnum<vi>, "App.Kind"=w353:T5)  [unwired: 2 in, 1 out]
        n174 = control-ref of="Current VI Reference"() -> (w348:refnum<vi>)
        n175 = Not(x=w354) -> (.not. x?=w351:bool)
        n176 = Equal?(x=w353, y=T5."Run Time System" ("Application:Kind")) -> (x = y?=w350:bool)
        n177 = Unbundle By Name(w347) -> ("status"=w346:bool)
        n178 = Not(x=w346) -> (.not. x?=w344:bool)
        n179 = Or(x=w351, y=w350) -> (x .or. y?=w342:bool)
        n180 = Or(x=w342, y=w344) -> (x .or. y?=w341:bool)
        n181 = Bundle By Name(cluster=w349, "Core.Current VI Reference"=w348, "Core.Close Panel on Exit?"=w341, "Core.NI.LV.Dialog namespace"=w344, "Core.Menu Launch:App"=w345, "Core.Local App"=w343) -> (w356:T10)
        n182 = call <vilib>:"Add State(s) to Queue__jki_lib_state_machine.vi"("State(s) in (\"\")"=w358) -> ("States Out"=w357:string)  [unwired: 14 in]
      }
      frame "Error Handler" {
        # "Handle any errors here.\nYou can also output any states to clean-up after errors occur"
        # "Clear error"
        n183 = Unbundle By Name(w360) -> ("code"=w363:i32)
        n184 = Unbundle By Name(w365) -> ("Errors"=w364:T11)
        n185 = for {
          tunnel: w364 -> [w381] mode=indexing
          tunnel: w363 -> [w382]
          tunnel: [w381] -> w361
          tunnel: [w380] -> w362
          stop <- w380 stop-if-true
          n186 = Unbundle By Name(w381) -> ("code"=w383:i32)
          n187 = Equal?(x=w383, y=w382) -> (x = y?=w380:bool)
        }
        n188 = case shown="True" w362 {
          tunnel: w361 -> [_ w379]
          tunnel: w360 -> [w370 _]
          tunnel: ["/* Post Error States" w375] -> w359
          frame False {
            # "Unhandled Error -- Display it"
            n189 = call <vilib>:"General Error Handler.vi"("error in (no error)"=w370) -> ()  [unwired: 1 in, 14 out]
          }
          frame True {
            # "Existing error code: look in the file for description\nand display it.\n\nIf error is critical, exit safely. Otherwise clear error and continue."
            n190 = Unbundle By Name(w379) -> ("Critical"=w378:bool, "Long"=w373:string, "code"=w374:i32)  [unwired: 1 out]
            n191 = Format Into String(format string="Error %d.\n\n%s", w374, w373) -> (resulting string=w372:string)  [unwired: 2 in, 1 out]
            n192 = One Button Dialog(message=w372) -> ()  [unwired: 2 out]
            n193 = Select(t="Macro: Exit", s=w378, f="/* Post Error States") -> (s? t:f=w375:string)
          }
        }
        n194 = call <vilib>:"Add State(s) to Queue__jki_lib_state_machine.vi"("State(s) in Front (\"\")"=w359, "State(s) in (\"\")"=w368) -> ("States Out"=w367:string)  [unwired: 13 in]
      }
      frame "Error" {
        # "Add an error code to the queue.\n(Will be processed by Error Handler case)"
        n195 = Decimal String To Number(string=w391, default (0L)=0 ("default (0 I32)")) -> (number=w385:i32)  [unwired: 2 out]
        n196 = Unbundle By Name(w390) -> ("Errors"=w386:T11)
        n197 = for {
          tunnel: w386 -> [w398] mode=indexing
          tunnel: w385 -> [w395]
          tunnel: [w394] -> w384
          stop <- w396 stop-if-true
          n198 = Unbundle By Name(w398) -> ("Short"=w394:string, "code"=w397:i32)
          n199 = Equal?(x=w397, y=w395) -> (x = y?=w396:bool)
        }
        n200 = Bundle By Name(cluster=errorcluster {"status"=TRUE, "code"=0, "source"=""} ("error out"), "source"=w384, "code"=w385) -> (w387:errorcluster)
        n201 = call <vilib>:"Add State(s) to Queue__jki_lib_state_machine.vi"("State(s) in (\"\")"=w393) -> ("States Out"=w392:string)  [unwired: 14 in]
      }
      frame "Exit" {
        # "Do not put any code in this frame.\n(No errors that occur here will be handled.)"
        n202 = call <vilib>:"Add State(s) to Queue__jki_lib_state_machine.vi"("State(s) in (\"\")"=w403) -> ("States Out"=w402:string)  [unwired: 14 in]
      }
      frame "---------- Data ----------" {
        # "Do not put any code in this frame.\n(It is a separator no-op. You can make a copy of this frame to create a new Data frame)"
        n203 = call <vilib>:"Add State(s) to Queue__jki_lib_state_machine.vi"("State(s) in (\"\")"=w407) -> ("States Out"=w406:string)  [unwired: 14 in]
      }
      frame "Data: Initialize" {
        w408 = cluster{"Icon source":path} {"Icon source"=path ""}  # Source
        w410 = cluster{"fade":u32, "droplabel":bool} {"fade"=750, "droplabel"=FALSE}  # config
        w411 = T12 {"Action"=4, "Orientations"=14, "Icon png"=path "", "Control Text"="", "Style"=0, "Text Color"=0, "Scale"=1.0, "Close afterwards"=FALSE}  # last state
        w409 = path ""  # file in tmp dir
        w413 = T11 []  # Errors
        w414 = refnum<class "Control.lvclass"> refnum  # Control
        w415 = T13 {"Current VI Reference"=refnum, "Close Panel on Exit?"=FALSE, "NI.LV.Dialog namespace"=FALSE, "Menu Launch:App"=refnum, "Local App"=refnum}  # Core
        # "Initialize the shift-register data, here.\n(data names are defined by what you wire into the bundle function)"
        n204 = Bundle("Core"=w415, "Control"=w414, "Errors"=w413, "user events"=w412, "last state"=w411, "config"=w410, "file in tmp dir"=w409, "Source"=w408) -> (w417:T10)  [unwired: 1 out]
        n205 = call <vilib>:"Add State(s) to Queue__jki_lib_state_machine.vi"("State(s) in (\"\")"=w419) -> ("States Out"=w418:string)  [unwired: 14 in]
      }
      frame "Data: Cleanup" {
        # "If not found in config.ini file, then set to default value."
        # "Cleanup any data and references, here.\n(this is called automatically, by the Macro: Exit)"
        n206 = Unbundle By Name(w437) -> ("Core.Current VI Reference"=w439:refnum<vi>)
        n207 = Unregister For Events(event registration refnum=w436) -> ()  [unwired: 1 in, 1 out]
        n208 = Close Reference(reference=w439, error in (no error)=w438) -> (error out=w427:errorcluster)
        n209 = call <userlib>:"Current VI's Path__ogtk.vi"() -> ("Current VI's Path (+ Relative)"=w432:path)  [unwired: 1 out]
        n210 = call <userlib>:"Current VIs Parent Directory__ogtk.vi"("Relative path (.)"=path "config.ini") -> ("Parent Directory (+ Relative)"=w433:path)  [unwired: 4 out]
        n211 = call-poly <userlib>:"Strip Path__ogtk.vi"("path"=w432) -> ("name"=w421:string)  [unwired: 1 out]
        n212 = call <vilib>:"Open Config Data (compatibility).vi"("error in (no error)"=w427, "configuration file path"=w433) -> ("error out"=w430:errorcluster, "refnum"=w431:T14)  [unwired: 7 in, 1 out]
        n213 = call-poly <vilib>:"Read Key.vi"("section"=w421, "error in (no error)"=w430, "default value"="750", "key"="fade", "refnum"=w431) -> ("error out"=w422:errorcluster, "found?"=w420:bool, "refnum out"=w423:T14)  [unwired: 1 in, 3 out]
        n214 = case shown="False" w420 {
          tunnel: [w448 w450] -> w425
          tunnel: [w447 w449] -> w424
          tunnel: w423 -> [w446 w450]
          tunnel: w422 -> [w445 w449]
          tunnel: w421 -> [w444 _]
          frame False {
            n215 = call-poly <vilib>:"Write Key.vi"("section"=w444, "error in (no error)"=w445, "value"="750", "key"="fade", "refnum"=w446) -> ("error out"=w447:errorcluster, "refnum out"=w448:T14)  [unwired: 1 in, 4 out]
          }
          frame True {
          }
        }
        n216 = call <vilib>:"Close Config Data.vi"("error in (no error)"=w424, "refnum"=w425) -> ("error out"=w426:errorcluster)  [unwired: 1 in, 8 out]
        n217 = call <vilib>:"Add State(s) to Queue__jki_lib_state_machine.vi"("State(s) in Front (\"\")"="" ("State(s) in Front (\"\")"), "State(s) in (\"\")"=w441) -> ("States Out"=w440:string)  [unwired: 13 in]
      }
      frame "---------- UI ----------" {
        # "Do not put any code in this frame.\n(It is a separator no-op. You can make a copy of this frame to create a new UI frame)"
        n218 = call <vilib>:"Add State(s) to Queue__jki_lib_state_machine.vi"("State(s) in (\"\")"=w454) -> ("States Out"=w453:string)  [unwired: 14 in]
      }
      frame "UI: Initialize" {
        # "Initialize the VI's behavior"
        # "Initialize the User Interface, here.\n(this is called automatically, by the Macro: Init)"
        n219 = Unbundle By Name(w457) -> ("Core.Current VI Reference"=w463:refnum<vi>)
        n220 = property class="VI"(reference=w463, "Front Panel.ShowMenuBar"=TRUE ("Front Panel Window:Show Menu Bar"), "Front Panel.TitleBarVis"=TRUE ("Front Panel Window:Show Menu Bar"), "Front Panel.Minimizeable"=TRUE ("Front Panel Window:Show Menu Bar"), "Front Panel.Resizeable"=FALSE ("Front Panel Window:Show Menu Bar"), "Front Panel.Closeable"=TRUE ("Front Panel Window:Show Menu Bar")) -> ()  [unwired: 1 in, 2 out]
        n221 = call <vilib>:"Add State(s) to Queue__jki_lib_state_machine.vi"("State(s) in Front (\"\")"="UI: Read Config\nUI: Transparency >> TRUE\nUI: FadeIn\nControl: Read error list\nUI: List Projects\nUI: List Open FPs" ("State(s) in Front (\"\")"), "State(s) in (\"\")"=w465) -> ("States Out"=w464:string)  [unwired: 13 in]
      }
      frame "UI: Read Config" {
        n222 = Unbundle By Name(w477) -> ("last state"=w472:T12, "config"=w479:cluster{"fade":u32, "droplabel":bool})
        n223 = call <userlib>:"Current VIs Parent Directory__ogtk.vi"("Relative path (.)"=path "config.ini") -> ("Parent Directory (+ Relative)"=w483:path)  [unwired: 4 out]
        n224 = call <vilib>:"Open Config Data (compatibility).vi"("error in (no error)"=w481, "configuration file path"=w483) -> ("error out"=w489:errorcluster, "refnum"=w486:T14)  [unwired: 7 in, 1 out]
        n225 = call <userlib>:"Current VI's Path__ogtk.vi"() -> ("Current VI's Path (+ Relative)"=w482:path)  [unwired: 1 out]
        n226 = call-poly <userlib>:"Strip Path__ogtk.vi"("path"=w482) -> ("name"=w485:string)  [unwired: 1 out]
        n227 = call <userlib>:"Set Data Name__ogtk.vi"("error in (no error)"=w489, "Data Name"=w485, "Data"=w479) -> ("error out"=w488:errorcluster, "Renamed Data"=w487:variant)  [unwired: 7 out]
        n228 = call <userlib>:"Read INI Cluster__ogtk.vi"("error in (no error)"=w488, "INI Fomatted Cluster Type"=w487, "refnum"=w486) -> ("error out"=w470:errorcluster, "INI Fomatted Cluster"=w490:variant, "dup refnum"=w468:T14)  [unwired: 6 out]
        n229 = Variant To Data(type=w479, Variant=w490) -> (data=w478:cluster{"fade":u32, "droplabel":bool})  [unwired: 1 in, 1 out]
        n230 = call <userlib>:"Set Data Name__ogtk.vi"("error in (no error)"=w470, "Data Name"="last state", "Data"=w472) -> ("error out"=w474:errorcluster, "Renamed Data"=w475:variant)  [unwired: 7 out]
        n231 = call <userlib>:"Read INI Cluster__ogtk.vi"("error in (no error)"=w474, "INI Fomatted Cluster Type"=w475, "refnum"=w468) -> ("error out"=w469:errorcluster, "INI Fomatted Cluster"=w473:variant, "dup refnum"=w467:T14)  [unwired: 6 out]
        n232 = Variant To Data(type=w472, Variant=w473) -> (data=w471:T12)  [unwired: 1 in, 1 out]
        n233 = Bundle By Name(cluster=w477, "last state"=w471, "config"=w478) -> (w476:T10)
        n234 = call <vilib>:"Close Config Data.vi"("error in (no error)"=w469, "refnum"=w467) -> ("error out"=w480:errorcluster)  [unwired: 1 in, 8 out]
        n235 = call <vilib>:"Add State(s) to Queue__jki_lib_state_machine.vi"("State(s) in (\"\")"=w492) -> ("States Out"=w491:string)  [unwired: 14 in]
      }
      frame "UI: Transparency" {
        # "if error ==> opaque"
        # "Initialize the User Interface, here.\n(this is called automatically, by the Macro: Init)"
        n236 = Unbundle By Name(w504) -> ("Core.Current VI Reference"=w503:refnum<vi>)
        n237 = Scan From String(format string="%s", input string=w502, default 1=FALSE) -> (error out=w496:errorcluster, output 1=w499:bool)  [unwired: 2 in, 2 out]
        n238 = Select(t=0, s=w496, f=100) -> (s? t:f=w493:i32)
        n239 = call <vilib>:"UI.SetTransparency__lava_lib_ui_tools.vi"("error in"=w498, "Run VI Transparently (T)"=w499, "Variant (%)"=w493, "VI Reference (calling VI)"=w503) -> ("error out"=w497:errorcluster)  [unwired: 7 out]
        n240 = call <vilib>:"Add State(s) to Queue__jki_lib_state_machine.vi"("State(s) in (\"\")"=w506) -> ("States Out"=w505:string)  [unwired: 14 in]
      }
      frame "UI: FadeIn" {
        # "Input is variant: \n\naccepts any numerics or string (%d format)"
        # "Initialize the User Interface, here.\n(this is called automatically, by the Macro: Init)"
        n241 = Unbundle By Name(w511) -> ("Core.Current VI Reference"=w510:refnum<vi>, "config.fade"=w507:u32)
        n242 = call <vilib>:"UI.FadeIn__lava_lib_ui_tools.vi"("error in"=w509, "Variant (ms)"=w507, "VI Reference (calling VI)"=w510) -> ("error out"=w508:errorcluster)  [unwired: 1 in, 7 out]
        n243 = call <vilib>:"Add State(s) to Queue__jki_lib_state_machine.vi"("State(s) in (\"\")"=w513) -> ("States Out"=w512:string)  [unwired: 14 in]
      }
      frame "UI: FadeOut" {
        # "Input is variant: \n\naccepts any numerics or string (%d format)"
        # "Initialize the User Interface, here.\n(this is called automatically, by the Macro: Init)"
        n244 = Unbundle By Name(w518) -> ("Core.Current VI Reference"=w517:refnum<vi>, "config.fade"=w514:u32)
        n245 = call <vilib>:"UI.FadeOut__lava_lib_ui_tools.vi"("error in"=w516, "Variant (ms)"=w514, "VI Reference (calling VI)"=w517) -> ("error out"=w515:errorcluster)  [unwired: 1 in, 7 out]
        n246 = call <vilib>:"Add State(s) to Queue__jki_lib_state_machine.vi"("State(s) in (\"\")"=w520) -> ("States Out"=w519:string)  [unwired: 14 in]
      }
      frame "UI: Cursor Set" {
        # "Argument"
        # "Set and Unset Cursor Busy.\n(Usage: \"UI: Cursor Set >> Busy|Idle\")"
        n247 = case shown="\"Idle\", Default" w521 {
          tunnel: w523 -> [w528 w530]
          tunnel: [w527 w529] -> w522
          frame "Idle", Default {
            n248 = call <vilib>:"Unset Busy.vi"("error in (no error)"=w528) -> ("error out"=w527:errorcluster)  [unwired: 1 in, 9 out]
          }
          frame "Busy" {
            n249 = call <vilib>:"Set Busy.vi"("error in (no error)"=w530) -> ("error out"=w529:errorcluster)  [unwired: 3 in, 7 out]
          }
        }
        n250 = call <vilib>:"Add State(s) to Queue__jki_lib_state_machine.vi"("State(s) in (\"\")"=w526) -> ("States Out"=w525:string)  [unwired: 14 in]
      }
      frame "UI: Front Panel State" {
        # "Argument"
        # "Set Front Panel Open or Closed\n(Usage: \"UI: Front Panel State >> Open|Close\")"
        n251 = Unbundle By Name(w533) -> ("Core.Current VI Reference"=w532:refnum<vi>)
        n252 = case shown="\"Open\", Default" w531 {
          tunnel: w535 -> [w541 w554]
          tunnel: [w543 w555] -> w534
          tunnel: w532 -> [w542 w552]
          frame "Open", Default {
            n253 = property class="VI"(reference=w542, error in=w541) -> (reference out=w539:refnum<vi>, error out=w540:errorcluster, "Front Panel.Open"=w538:bool)
            n254 = case shown="False" w538 {
              tunnel: [w546 w549] -> w543
              tunnel: w540 -> [w545 w549]
              tunnel: w539 -> [w544 _]
              frame False {
                n255 = invoke class="VI" method="FP.Open"(reference=w544, error in=w545, "Activate"=TRUE, "State"=T6."Standard") -> (error out=w546:errorcluster)  [unwired: 1 in, 4 out]
              }
              frame True {
              }
            }
          }
          frame "Close" {
            n256 = property class="VI"(reference=w552, error in=w554) -> (reference out=w551:refnum<vi>, error out=w553:errorcluster, "Front Panel.Open"=w550:bool)
            n257 = case shown="True" w550 {
              tunnel: [w556 w559] -> w555
              tunnel: w553 -> [w556 w558]
              tunnel: w551 -> [_ w557]
              frame False {
              }
              frame True {
                n258 = invoke class="VI" method="FP.Close"(reference=w557, error in=w558) -> (error out=w559:errorcluster)  [unwired: 1 in, 2 out]
              }
            }
          }
        }
        n259 = call <vilib>:"Add State(s) to Queue__jki_lib_state_machine.vi"("State(s) in (\"\")"=w537) -> ("States Out"=w536:string)  [unwired: 14 in]
      }
      frame "UI: List Projects" {
        # "List all projects currently in memory in the same application instance as the caller of this utility."
        n260 = Unbundle By Name(w561) -> ("Core.Menu Launch:App"=w563:refnum<vi>, "Core.NI.LV.Dialog namespace"=w564:bool, "Core.Local App"=w562:refnum<vi>)
        n261 = Select(t=w563, s=w564, f=w562) -> (s? t:f=w560:refnum<vi>)
        n262 = property class="App"(reference=w560) -> ("Project"=w566:refnum<vi>[])  [unwired: 1 in, 2 out]
        n263 = for {
          tunnel: [w579] -> w567 mode=indexing
          tunnel: w566 -> [w578] mode=indexing
          tunnel: [w577] -> w565 mode=indexing
          n264 = property class="Project"(reference=w578) -> (reference out=w577:refnum<vi>, "Name"=w579:string)  [unwired: 1 in, 1 out]
        }
        n265 = Array Size(array=w566) -> (size(s)=w569:i32)
        n266 = Greater Than 0?(x=w569) -> (x > 0?=w572:bool)
        n267 = local write "Add to Project"(w572) -> ()
        n268 = Close Reference(reference=w565) -> ()  [unwired: 1 in, 1 out]
        n269 = Select(t=u8 0 ("Disabled"), s=w572, f=u8 2 ("Disabled")) -> (s? t:f=w573:u8)
        n270 = property on="Projects" class="Ring (strict)"("Strings []"=w567, "Value"=0, "Disabled"=w573) -> ()  [unwired: 2 in, 2 out]
        n271 = property on="Add to Project" class="Bool (strict)"("Disabled"=w573) -> ()  [unwired: 2 in, 2 out]
        n272 = call <vilib>:"Add State(s) to Queue__jki_lib_state_machine.vi"("State(s) in (\"\")"=w576) -> ("States Out"=w575:string)  [unwired: 14 in]
      }
      frame "UI: List Open FPs" {
        w594 = u16 0 items=[""] ("Front Panels")
        # "Disable \"Drop on FP\" option\nif no idle FPs are opened."
        # "keep only Idle front panels to remove this VI,  \"probe VIs\" and\nVIs that are not in a state for scripting to work."
        # "ADAPTED FROM: \nList Open Front Panels.vi\nTO LIST ALL OPEN FRONT PANELS IN THE SELECTED APPLICATION INSTANCE\n\nReturns an array of the names of all VIs in memory whose front panels are open.\n\nPlease visit http://www.OpenG.org to learn about the\nOpen Source LabVIEW software movement.\n\nNOTICE -- YOU MUST LEAVE THIS NOTICE IN PLACE.  PER THE TERMS OF THE LICENSE BELOW, YOU MAY SUBLICENSE THIS SOFTWARE \nIN ANY WAY THAT DOES NOT CONFLICT WITH THIS LICENSE.\n\n### BSD License (http://www.opensource.org/licenses/bsd-license.php) Begin ###\n \nCopyright (c) 2002, Jim Kring <jim@jimkring.com>\n\nAll rights reserved.\n\nRedistribution and use in source and binary forms, with or without modification, are permitted provided that the following conditions are met:\n\n    * Redistributions of source code must retain the above copyright notice, this list of conditions and the following disclaimer.\n    * Redistributions in binary form must reproduce the above copyright notice, this list of conditions and the following disclaimer in the \n       documentation and/or other materials provided with the distribution.\n    * Neither the name of SciWare, James Kring, Inc., nor the names of its contributors may be used to endorse or promote products derived \n       from this software without specific prior written permission.\n\nTHIS SOFTWARE IS PROVIDED BY THE COPYRIGHT HOLDERS AND CONTRIBUTORS \"AS IS\" AND ANY EXPRESS OR IMPLIED WARRANTIES, \nINCLUDING, BUT NOT LIMITED TO, THE IMPLIED WARRANTIES OF MERCHANTABILITY AND FITNESS FOR A PARTICULAR PURPOSE ARE \nDISCLAIMED. IN NO EVENT SHALL THE COPYRIGHT OWNER OR CONTRIBUTORS BE LIABLE FOR ANY DIRECT, INDIRECT, INCIDENTAL,\n SPECIAL, EXEMPLARY, OR CONSEQUENTIAL DAMAGES (INCLUDING, BUT NOT LIMITED TO, PROCUREMENT OF SUBSTITUTE GOODS OR \nSERVICES; LOSS OF USE, DATA, OR PROFITS; OR BUSINESS INTERRUPTION) HOWEVER CAUSED AND ON ANY THEORY OF LIABILITY, \nWHETHER IN CONTRACT, STRICT LIABILITY, OR TORT (INCLUDING NEGLIGENCE OR OTHERWISE) ARISING IN ANY WAY OUT OF THE USE \nOF THIS SOFTWARE, EVEN IF ADVISED OF THE POSSIBILITY OF SUCH DAMAGE.\n\n### BSD License End ###"
        n273 = Unbundle By Name(w584) -> ("Core.Menu Launch:App"=w582:refnum<vi>, "Core.NI.LV.Dialog namespace"=w583:bool, "Core.Local App"=w581:refnum<vi>)
        n274 = Select(t=w582, s=w583, f=w581) -> (s? t:f=w585:refnum<vi>)
        n275 = property class="App"(reference=w585) -> (reference out=w586:refnum<vi>, "Application:All VIs In Memory"=w588:string[])  [unwired: 1 in, 1 out]
        n276 = for {
          tunnel: w588 -> [w608] mode=indexing
          shift-right: [w606] -> w580
          shift-left: string[] [] ("Application:All VIs In Memory") -> [w607]
          tunnel: w586 -> [w604]
          tunnel: [w598] -> _ mode=indexing
          n277 = Open VI Reference(application reference (local)=w604, vi path=w608, options=2) -> (vi reference=w612:refnum<vi>, error out=w611:errorcluster)  [unwired: 1 in, 2 out]
          n278 = property class="VI"(reference=w612, error in=w611) -> (reference out=w610:refnum<vi>, error out=w609:errorcluster, "Front Panel Window:Open"=w600:bool, "Exec.State"=w603:T7)
          n279 = Equal?(x=w603, y=T7."Idle" ("Execution:State")) -> (x = y?=w601:bool)
          n280 = And(x=w600, y=w601) -> (x .and. y?=w599:bool)
          n281 = case shown="True" w599 {
            tunnel: w608 -> [_ w616]
            tunnel: w607 -> [w613 w615]
            tunnel: [w613 w614] -> w606
            frame False {
            }
            frame True {
              n282 = Build Array (concatenate)(w615, w616) -> (w614:string[])
            }
          }
          n283 = Close Reference(reference=w610, error in (no error)=w609) -> (error out=w598:errorcluster)
        }
        n284 = Array Size(array=w580) -> (size(s)=w589:i32)
        n285 = Greater Than 0?(x=w589) -> (x > 0?=w592:bool)
        n286 = Select(t=u8 0 ("Disabled"), s=w592, f=u8 2 ("Disabled")) -> (s? t:f=w593:u8)
        n287 = property on="Front Panels" class="Ring (strict)"("Value"=w594, "Strings []"=w580, "Disabled"=w593) -> ()  [unwired: 2 in, 2 out]
        n288 = property on="Drop on Front Panel" class="Bool (strict)"("Value"=w592, "Disabled"=w593) -> ()  [unwired: 2 in, 2 out]
        n289 = call <vilib>:"Add State(s) to Queue__jki_lib_state_machine.vi"("State(s) in (\"\")"=w597) -> ("States Out"=w596:string)  [unwired: 14 in]
      }
      frame "---------- Macro ----------" {
        # "Do not put any code in this frame.\n(It is a separator no-op. You can make a copy of this frame to create a new Macro frame)"
        n290 = call <vilib>:"Add State(s) to Queue__jki_lib_state_machine.vi"("State(s) in (\"\")"=w620) -> ("States Out"=w619:string)  [unwired: 14 in]
      }
      frame "Macro: Initialize" {
        w621 = "Data: Initialize\nInitialize Core Data\nUI: Initialize\nUI: Front Panel State >> Open\nControl: Init"  # Data: Initialize Initialize Core Data UI: Initialize UI: Front Panel State >> Open Control: Init
        # "Initialization Macro\n(This is called once, when the VI starts)"
        n291 = call <vilib>:"Add State(s) to Queue__jki_lib_state_machine.vi"("State(s) in Front (\"\")"=w621, "State(s) in (\"\")"=w625) -> ("States Out"=w624:string)  [unwired: 13 in]
      }
      frame "Macro: Exit" {
        # "Exit Macro\n(This is called once, when the VI exits)"
        n292 = Unbundle By Name(w628) -> ("Core.Close Panel on Exit?"=w634:bool)  [unwired: 1 out]
        n293 = Select(t="UI: Front Panel State >> Close", s=w634, f="") -> (s? t:f=w631:string)
        n294 = call <vilib>:"Add State(s) to Queue__jki_lib_state_machine.vi"("State(s) in Front (\"\")"="UI: FadeOut", "State(s) in (\"\")"=w631, "State(s) at Back (\"\")"="Data: Cleanup\nExit") -> ("States Out"=w629:string)  [unwired: 12 in]
        n295 = call <vilib>:"Add State(s) to Queue__jki_lib_state_machine.vi"("State(s) in Front (\"\")"=w629, "State(s) in (\"\")"=w636) -> ("States Out"=w635:string)  [unwired: 13 in]
      }
      frame "---------- Control ----------" {
        # "Template Separator\n(You can make a copy of, or modify, this frame)"
        n296 = call <vilib>:"Add State(s) to Queue__jki_lib_state_machine.vi"("State(s) in (\"\")"=w640) -> ("States Out"=w639:string)  [unwired: 14 in]
      }
      frame "Preview" {
        # "Resize and Display"
        # "Add the other states"
        # "Get first state"
        # "Generate a preview in the right-end side of the interface.\nIf many button states are found, then they will be concatenated to a single picture."
        n297 = Unbundle By Name(w645) -> ("Control"=w646:refnum<class "Control.lvclass">)
        n298 = call-dynamic "Preview Control States.vi"("Control in"=w646) -> ("States preview"=w647:picture[], "Control out"=w643:refnum<class "Control.lvclass">)  [unwired: 1 in, 8 out]
        n299 = Delete From Array(array=w647, length=1, index=0) -> (deleted portion=w652:picture[], array with subset deleted=w653:picture[])
        n300 = Index Array(array=w652) -> (element=w649:picture)  [unwired: 1 in]
        n301 = call <vilib>:"Picture to Pixmap.vi"("Background Color"=u32 16448250 ("Color Box"), "depth"=24, "picture"=w649) -> ("image data"=w657:T15)  [unwired: 1 in, 7 out]
        n302 = for {
          tunnel: w653 -> [w669] mode=indexing
          shift-right: [w665] -> w654
          shift-left: w657 -> [w664]
          n303 = call <vilib>:"Picture to Pixmap.vi"("Background Color"=u32 16448250 ("Color Box"), "picture"=w669) -> ("image data"=w663:T15)  [unwired: 2 in, 7 out]
          n304 = call <vilib>:"Unflatten Pixmap.vi"("image data"=w664) -> ("24-bit pixmap"=w668:u32[][])  [unwired: 10 out]
          n305 = call <vilib>:"Unflatten Pixmap.vi"("image data"=w663) -> ("24-bit pixmap"=w667:u32[][])  [unwired: 10 out]
          n306 = Build Array (concatenate)(w668, w667) -> (w666:u32[][])
          n307 = call <vilib>:"Flatten Pixmap.vi"("24-bit pixmap"=w666) -> ("image data"=w665:T15)  [unwired: 5 in, 5 out]
        }
        n308 = control-ref of="Controls preview"() -> (w642:refnum<vi>)
        n309 = Unbundle By Name(w654) -> ("Rectangle"=w655:T16)
        n310 = call <vilib>:"Draw Flattened Pixmap.vi"("image data"=w654) -> ("new picture"=→"Controls preview":picture)  [unwired: 1 in, 7 out]
        n311 = call <vilib>:"RectSize.vi"("rect"=w655) -> ("point"=w656:cluster{"x":i16, "y":i16})
        n312 = Bundle By Name(cluster=w645, "Control"=w643) -> (w644:T10)
        n313 = property class="Pict"(reference=w642, "Draw Area Size"=w656) -> ()  [unwired: 1 in, 2 out]
        n314 = call <vilib>:"Add State(s) to Queue__jki_lib_state_machine.vi"("State(s) in (\"\")"=w661) -> ("States Out"=w660:string)  [unwired: 14 in]
      }
      frame "Control: Read error list" {
        # "Read the error list from the file."
        n315 = Unbundle By Name(w675) -> ("Control"=w680:refnum<class "Control.lvclass">, "Errors"=w671:T11)
        n316 = Index Array(array=w671) -> (element=w670:T17)  [unwired: 1 in]
        n317 = call <vilib>:"Get LV Class Path.vi"("object"=w680) -> ("error out"=w684:errorcluster, "class path"=w686:path)  [unwired: 1 in, 8 out]
        n318 = while {
          shift-right: [w712] -> w687
          shift-left: w686 -> [w714]
          tunnel: w684 -> [_]
          stop <- w716 stop-if-true
          # "Extracted from OpenG: \n\"Current VI Parent Dir\""
          n319 = call-poly <userlib>:"Strip Path__ogtk.vi"("path"=w714) -> ("stripped path"=w712:path)  [unwired: 1 out]
          n320 = File/Directory Info(path=w712) -> (directory=w717:bool)  [unwired: 1 in, 6 out]
          n321 = Not A Number/Path/Refnum?(number/path/refnum=w714) -> (NaN/Path/Refnum?=w715:bool)
          n322 = Empty String/Path?(string/path=w714) -> (empty?=w713:bool)
          n323 = Compound Arithmetic op=OR(w717, w715, w713) -> (w716:bool)
        }
        n324 = Build Path(base path=w687, name or relative path="errors.txt") -> (appended path=w683:path)
        n325 = call <vilib>:"Open Config Data (compatibility).vi"("configuration file path"=w683) -> ("error out"=w682:errorcluster, "refnum"=w681:T14)  [unwired: 8 in, 1 out]
        n326 = call <vilib>:"Get Section Names.vi"("error in (no error)"=w682, "refnum"=w681) -> ("error out"=w679:errorcluster, "section names"=w672:string[], "refnum out"=w678:T14)  [unwired: 1 in, 6 out]
        n327 = for {
          shift-right: [w706] -> w677
          shift-left: w678 -> [w710]
          shift-right: [w707] -> w676
          shift-left: w679 -> [w711]
          tunnel: w672 -> [w700] mode=indexing
          tunnel: [w709] -> w673 mode=indexing
          tunnel: w670 -> [w708]
          n328 = Decimal String To Number(string=w700) -> (number=w691:i32)  [unwired: 3 out]
          n329 = call-poly <vilib>:"Read Key.vi"("section"=w700, "error in (no error)"=w711, "default value"=FALSE, "key"="Critical" ("name or relative path"), "refnum"=w710) -> ("error out"=w703:errorcluster, "value"=w692:bool, "refnum out"=w704:T14)  [unwired: 4 out]
          n330 = call-poly <vilib>:"Read Key.vi"("section"=w700, "error in (no error)"=w703, "default value"="", "key"="Long" ("name or relative path"), "refnum"=w704) -> ("error out"=w702:errorcluster, "value"=w694:string, "refnum out"=w705:T14)  [unwired: 1 in, 3 out]
          n331 = call-poly <vilib>:"Read Key.vi"("section"=w700, "error in (no error)"=w702, "default value"="", "key"="Short" ("name or relative path"), "refnum"=w705) -> ("error out"=w707:errorcluster, "value"=w695:string, "refnum out"=w706:T14)  [unwired: 1 in, 3 out]
          n332 = Bundle(cluster=w708, "code"=w691, "Short"=w695, "Long"=w694, "Critical"=w692) -> (w709:T17)
        }
        n333 = Bundle By Name(cluster=w675, "Errors"=w673) -> (w674:T10)
        n334 = call <vilib>:"Add State(s) to Queue__jki_lib_state_machine.vi"("State(s) in (\"\")"=w690) -> ("States Out"=w689:string)  [unwired: 14 in]
        n335 = call <vilib>:"Close Config Data.vi"("error in (no error)"=w676, "refnum"=w677) -> ()  [unwired: 1 in, 9 out]
      }
      frame "Control: Save Temp Control" {
        # "Create a temporary filename for the control to be saved in."
        n336 = Unbundle By Name(w727) -> ("Control"=w725:refnum<class "Control.lvclass">)
        n337 = call-dynamic "Read Target path ctl.vi"("Control in"=w725) -> ("Target path (.ctl)"=w724:path, "Control out"=w721:refnum<class "Control.lvclass">)  [unwired: 1 in, 8 out]
        n338 = call <userlib>:"Temporary Filename__ogtk.vi"("pattern (lvtemp%d.tmp)"="temp_control_%d.ctl" ("pattern (all files)"), "sub directory"=path "control") -> ("file in tmp dir"=w718:path)  [unwired: 1 in, 4 out]
        n339 = call-dynamic "Create Control (to dir).vi"("Target Folder or .ctl"=w718, "Control in"=w721) -> ("Control out"=w722:refnum<class "Control.lvclass">)  [unwired: 1 in, 8 out]
        n340 = call-dynamic "Write Target path ctl.vi"("Target path (.ctl)"=w724, "Control in"=w722) -> ("Control out"=w723:refnum<class "Control.lvclass">)  [unwired: 1 in, 8 out]
        n341 = Bundle By Name(cluster=w727, "Control"=w723, "file in tmp dir"=w718) -> (w726:T10)
        n342 = call <vilib>:"Add State(s) to Queue__jki_lib_state_machine.vi"("State(s) in (\"\")"=w730) -> ("States Out"=w729:string)  [unwired: 14 in]
      }
      frame "Control: Prepare batch" {
        # "TO BE ADDED:\n\nWhen preparing for batch processing, launch a VI\nwith VI Server that will calculate the number of PNGs in the\ndirectory recursively while letting this utility run in parallel.\nOtherwise, if the number of files is huge, it could make the\nutility appear to hang indefinitely.\n\nTake only the first PNG for preview."
        n343 = Unbundle By Name(w735) -> ("Control"=w733:refnum<class "Control.lvclass">)
        n344 = disable-structure shown="Disabled" {
          disable-tunnel: "Icon source" -> [w740 _]
          disable-tunnel: "*.png" ("pattern") -> [w739 _]
          frame Disabled {
            n345 = call <userlib>:"List Directory Recursive__ogtk.vi"("pattern"=w739, "Path"=w740) -> ()  [unwired: 3 in, 7 out]
          }
          frame Enabled {
          }
        }
        n346 = Bundle By Name(cluster=w735, "Control"=w733) -> (w734:T10)
        n347 = call <vilib>:"Add State(s) to Queue__jki_lib_state_machine.vi"("State(s) in (\"\")"=w738) -> ("States Out"=w737:string)  [unwired: 14 in]
      }
      frame "Control: Save Control to Disk" {
        n348 = local read "Add to Project"() -> (w749:bool)
        n349 = Unbundle By Name(w759) -> ("Control"=w747:refnum<class "Control.lvclass">)
        n350 = case shown="True" w749 {
          tunnel: [w771 w777] -> w748
          frame False {
            n351 = Call Chain() -> (call chain=w776:string[])
            n352 = Reverse 1D Array(array=w776) -> (reversed array=w775:string[])
            n353 = Index Array(array=w775) -> (element=w774:string)  [unwired: 1 in]
            n354 = Open VI Reference(vi path=w774) -> (vi reference=w773:refnum<vi>)  [unwired: 1 in, 5 out]
            n355 = property class="VI"(reference=w773) -> ("Path"=w772:path)  [unwired: 1 in, 2 out]
            n356 = Strip Path(path=w772) -> (stripped path=w771:path)  [unwired: 1 out]
          }
          frame True {
            # "If \"Add to Project\" selected, then set start path to be the \nsame as the project's directory."
            n357 = property on="Projects" class="Ring (strict)"() -> ("Strings []"=w779:string[], "Value"=w778:u16)  [unwired: 2 in, 2 out]
            n358 = Index Array(array=w779, index=w778) -> (element=w780:string)
            n359 = call "Get project path.vi"("Project Name"=w780) -> ("Project path"=w777:path)
          }
        }
        n360 = local read "Control Text"() -> (w753:string)
        n361 = property on="Button Style" class="Ring (strict)"() -> ("Strings []"=w757:string[], "Value"=w756:u16)  [unwired: 2 in, 2 out]
        n362 = Index Array(array=w757, index=w756) -> (element=w755:string)
        n363 = Concatenate Strings(w755, "_" ("string"), w753, ".ctl" ("pattern (all files)")) -> (w750:string)
        n364 = call "File Dialog4"("start path"=w748, "default name"=w750, "error in"=w741, "pattern (all files)"="*.ctl") -> ("selected path"=w745:path, "cancelled"=w744:bool, "error out"=w743:errorcluster)  [unwired: 3 in, 6 out]
        n365 = case shown="False" w744 {
          tunnel: w747 -> [w766 w770]
          tunnel: [w768 w770] -> w746
          tunnel: w745 -> [w764 _]
          tunnel: w743 -> [w763 w769]
          tunnel: [w767 w769] -> w742
          frame False {
            n366 = call-dynamic "Write Target path ctl.vi"("error in (no error)"=w763, "Target path (.ctl)"=w764, "Control in"=w766) -> ("error out"=w762:errorcluster, "Control out"=w765:refnum<class "Control.lvclass">)  [unwired: 7 out]
            n367 = call-dynamic "Create Control (to dir).vi"("error in (no error)"=w762, "Target Folder or .ctl"=w764, "Control in"=w765) -> ("error out"=w767:errorcluster, "Control out"=w768:refnum<class "Control.lvclass">)  [unwired: 7 out]
          }
          frame True {
          }
        }
        n368 = Bundle By Name(cluster=w759, "Control"=w746) -> (w758:T10)
        n369 = call <vilib>:"Add State(s) to Queue__jki_lib_state_machine.vi"("State(s) in (\"\")"=w761) -> ("States Out"=w760:string)  [unwired: 14 in]
      }
      frame "Control: Add to FP" {
        w805 = refnum<vi> refnum  # Boolean
        # "Add to selected FP.\n\nTO ADD: \nCalculate best location to drop the control..."
        n370 = Unbundle By Name(w790) -> ("Control"=w799:refnum<class "Control.lvclass">, "Core.Menu Launch:App"=w787:refnum<vi>, "Core.NI.LV.Dialog namespace"=w788:bool, "Core.Local App"=w782:refnum<vi>)
        n371 = property on="Front Panels" class="Ring (strict)"(error in=w797) -> (error out=w785:errorcluster, "Strings []"=w801:string[])  [unwired: 1 in, 1 out]
        n372 = Index Array(array=w801, index="Front Panels") -> (element=w795:string)
        n373 = Select(t=w787, s=w788, f=w782) -> (s? t:f=w786:refnum<vi>)
        n374 = Unbundle By Name(w790) -> ("file in tmp dir"=w789:path, "config.droplabel"=w783:bool)
        n375 = Open VI Reference(application reference (local)=w786, vi path=w795, error in (no error)=w785) -> (vi reference=w796:refnum<vi>, error out=w806:errorcluster)  [unwired: 3 out]
        n376 = property class="VI"(reference=w796, error in=w806) -> (reference out=w802:refnum<vi>, error out=w803:errorcluster, "Panel"=w781:refnum<vi>)
        n377 = New VI Object(vi object class=w805, owner refnum=w781, position/next to=T8 {"Horizontal"=0, "Vertical"=0} ("relative position/next to refnum"), 6:w789, 8:w803) -> (object refnum=w794:refnum<vi>, 0:w793:errorcluster)  [unwired: 3 out]
        n378 = property class="Bool"(reference=w794, error in=w793, "Label.Visible"=w783) -> (reference out=w792:refnum<vi>, error out=w791:errorcluster)
        n379 = Close Reference(reference=w792, error in (no error)=w791) -> (error out=w784:errorcluster)
        n380 = Bundle By Name(cluster=w790, "Control"=w799) -> (w807:T10)
        n381 = Close Reference(reference=w802, error in (no error)=w784) -> (error out=w798:errorcluster)
        n382 = call <vilib>:"Add State(s) to Queue__jki_lib_state_machine.vi"("State(s) in (\"\")"=w809) -> ("States Out"=w808:string)  [unwired: 14 in]
      }
      frame "Control: Add to palette" {
        w820 = T18 -2 items=["Functions"=-1, "Controls"=-2] ("palette type")
        # "- Add the control to the palette selected. (Defaults to <user.lib>\\_LAVAcr\\CustomControls)"
        # "- Add to dir.mnu file located in <user.lib>\\_LAVAcr\\CustomControls"
        # "TO BE ADDED: \nSet the name to something meaningful (and unique)"
        n383 = Unbundle By Name(w839) -> ("Control"=w837:refnum<class "Control.lvclass">, "Core.Menu Launch:App"=w823:refnum<vi>, "Core.NI.LV.Dialog namespace"=w824:bool, "Core.Local App"=w822:refnum<vi>, "file in tmp dir"=w828:path)
        n384 = call-poly <userlib>:"Strip Path__ogtk.vi"("path"=w828) -> ("name"=w811:string)  [unwired: 1 out]
        n385 = call <userlib>:"User Library__ogtk.vi"("Relative path (.)"="Palette") -> ("User Library (+ Relative)"=w829:path)
        n386 = Select(t=w823, s=w824, f=w822) -> (s? t:f=w821:refnum<vi>)
        n387 = call <userlib>:"Create Dir if Non-Existant__ogtk.vi"("error in (no error)"=w832, "Directory Path"=w829) -> ("error out"=w833:errorcluster, "dup Directory Path"=w835:path)  [unwired: 1 in, 7 out]
        n388 = call-poly <userlib>:"Build Path__ogtk.vi"("name or relative path"=w811, "base path"=w835) -> ("appended path"=w836:path)
        n389 = call <userlib>:"User Library__ogtk.vi"("Relative path (.)"=path "_LAVAcr/CustomControls/dir.mnu") -> ("User Library (+ Relative)"=w827:path)
        n390 = call <userlib>:"Copy with Options__ogtk.vi"("error in (no error)"=w833, "target path"=w836, "source path"=w828) -> ("error out"=w826:errorcluster, "new path"=w816:path)  [unwired: 1 in, 6 out]
        n391 = call-poly <userlib>:"Strip Path Extension__ogtk.vi"("path"=w811) -> ("root"=w810:string)  [unwired: 1 out]
        n392 = call <vilib>:"Read Palette.vi"("application reference"=w821, "error in (no error)"=w826, "palette type"=w820, "palette path"=w827) -> ("palette data"=w817:T19, "duplicate palette path"=w825:path)  [unwired: 6 out]
        n393 = Unbundle By Name(w817) -> ("items"=w813:T21)
        n394 = Bundle By Name(cluster=T9 {"item path"=path "", "library path (.lvlib)"=path "", "use default lvlib palette"=FALSE, "short name"="", "place VI contents"=FALSE, "hide synchronized item"=FALSE, "reserve spot for synch item"=FALSE, "configure when placing VI contents"=FALSE} ("element"), "item path"=w816, "short name"=w810) -> (w814:T9)
        n395 = Build Array (concatenate)(w813, w814) -> (w812:T21)
        n396 = Bundle By Name(cluster=w817, "items"=w812) -> (w818:T19)
        n397 = call <vilib>:"Write Palette.vi"("application reference"=w821, "palette data"=w818, "palette type"=w820, "palette path"=w825) -> ("error out"=w819:errorcluster)  [unwired: 1 in, 6 out]
        n398 = Bundle By Name(cluster=w839, "Control"=w837) -> (w838:T10)
        n399 = invoke class="App" method="Refresh Palettes"(error in=w819) -> (error out=w831:errorcluster)  [unwired: 2 in, 2 out]
        n400 = call <vilib>:"Add State(s) to Queue__jki_lib_state_machine.vi"("State(s) in (\"\")"=w841) -> ("States Out"=w840:string)  [unwired: 14 in]
      }
      frame "Control: Add to Project" {
        # "If the file has not been added to disk, then copy the temp control to the\nproject directory with a meaningful name and add it to lvproj file."
        n401 = Unbundle By Name(w843) -> ("Core.Menu Launch:App"=w846:refnum<vi>, "Core.NI.LV.Dialog namespace"=w847:bool, "Core.Local App"=w845:refnum<vi>, "file in tmp dir"=w842:path)
        n402 = Unbundle By Name(w843) -> ("Control"=w870:refnum<class "Control.lvclass">)
        n403 = local read "Control Text"() -> (w850:string)
        n404 = property on="Button Style" class="Ring (strict)"() -> ("Strings []"=w854:string[], "Value"=w853:u16)  [unwired: 2 in, 2 out]
        n405 = call-dynamic "Read Target path ctl.vi"("error in (no error)"=w861, "Control in"=w870) -> ("error out"=w880:errorcluster, "Target path (.ctl)"=w858:path, "Control out"=w869:refnum<class "Control.lvclass">)  [unwired: 7 out]
        n406 = Index Array(array=w854, index=w853) -> (element=w852:string)
        n407 = Select(t=w846, s=w847, f=w845) -> (s? t:f=w844:refnum<vi>)
        n408 = Concatenate Strings(w852, "_" ("string"), w850, ".ctl" ("pattern (all files)")) -> (w848:string)
        n409 = call-poly <userlib>:"File Exists__ogtk.vi"("file path"=w858) -> ("is directory"=w863:bool, "exists"=w864:bool)  [unwired: 6 in]
        n410 = property on="Projects" class="Ring (strict)"() -> ("Strings []"=w867:string[], "Value"=w866:u16)  [unwired: 2 in, 2 out]
        n411 = Compound Arithmetic op=AND(invert w863, w864) -> (w859:bool)
        n412 = property class="App"(reference=w844, error in=w880) -> ("Project"=w878:refnum<vi>[])  [unwired: 2 out]
        n413 = Index Array(array=w867, index=w866) -> (element=w868:string)
        n414 = call "Get project path.vi"("Project Name"=w868) -> ("Project path"=w862:path)
        n415 = Index Array(array=w878, index="Projects") -> (element=w879:refnum<vi>)
        n416 = call-poly <userlib>:"Build Path__ogtk.vi"("name or relative path"=w848, "base path"=w862) -> ("appended path"=w881:path)
        n417 = property class="Project"(reference=w879) -> (reference out=w876:refnum<vi>, error out=w872:errorcluster, "My Computer"=w877:refnum<vi>)  [unwired: 1 in]
        n418 = Close Reference(reference=w876, error in (no error)=w872) -> (error out=w857:errorcluster)
        n419 = case shown="False" w859 {
          tunnel: w881 -> [w889 _]
          tunnel: w842 -> [w888 _]
          tunnel: [w887 w890] -> w855
          tunnel: [w886 w891] -> w860
          tunnel: w858 -> [_ w891]
          tunnel: w857 -> [w885 w890]
          frame False {
            n420 = call <userlib>:"Copy with Options__ogtk.vi"("error in (no error)"=w885, "target path"=w889, "source path"=w888) -> ("error out"=w887:errorcluster, "new path"=w886:path)  [unwired: 1 in, 6 out]
          }
          frame True {
          }
        }
        n421 = invoke class="TargetItem" method="AddFile"(reference=w877, error in=w855, "Path"=w860) -> (reference out=w875:refnum<vi>, error out=w873:errorcluster, "AddFile"=w874:refnum<vi>)  [unwired: 1 in, 1 out]
        n422 = Bundle By Name(cluster=w843, "Control"=w869) -> (w882:T10)
        n423 = Close Reference(reference=w875, error in (no error)=w873) -> (error out=w871:errorcluster)
        n424 = call <vilib>:"Add State(s) to Queue__jki_lib_state_machine.vi"("State(s) in (\"\")"=w884) -> ("States Out"=w883:string)  [unwired: 14 in]
        n425 = Close Reference(reference=w874, error in (no error)=w871) -> (error out=w856:errorcluster)
      }
      frame "Control: Delete Temp Control" {
        # "Delete the temporary control file."
        n426 = Unbundle By Name(w901) -> ("Control"=w899:refnum<class "Control.lvclass">, "file in tmp dir"=w892:path)
        n427 = call <userlib>:"Delete Recursive__ogtk.vi"("Ignore Read-Only? (FALSE)"=FALSE, "Path"=w892) -> ("error out"=w897:errorcluster)  [unwired: 2 in, 7 out]
        n428 = Select(t="Error >> 7002" ("pattern (all files)"), s=w897, f="") -> (s? t:f=w894:string)
        n429 = Bundle By Name(cluster=w901, "Control"=w899, "file in tmp dir"=path "") -> (w900:T10)
        n430 = call <vilib>:"Add State(s) to Queue__jki_lib_state_machine.vi"("State(s) in Front (\"\")"=w894, "State(s) in (\"\")"=w904) -> ("States Out"=w903:string)  [unwired: 13 in]
      }
      frame "Control: Init" {
        n431 = call "Init_Control.vi"("error in (no error)"=w912) -> ("error out"=w916:errorcluster, "App.SaveVersions"=w913:string[], "Styles strings"=w909:string[], "Control out"=w910:refnum<class "Control.lvclass">)  [unwired: 7 out]
        n432 = Empty Array?(array=w909) -> (empty?=w908:bool)
        n433 = property on="Button Style" class="Ring (strict)"(error in=w916, "Strings []"=w909, "Value"=0) -> (error out=w914:errorcluster)  [unwired: 1 in, 1 out]
        n434 = Select(t="Error >> 7000", s=w908, f="Control: Read Config") -> (s? t:f=w905:string)
        n435 = Bundle By Name(cluster=w919, "Control"=w910) -> (w918:T10)
        n436 = property on="Save for version" class="Ring (strict)"(error in=w914, "Strings []"=w913, "Value"=0) -> (error out=w911:errorcluster)  [unwired: 1 in, 1 out]
        n437 = call <vilib>:"Add State(s) to Queue__jki_lib_state_machine.vi"("State(s) in Front (\"\")"=w905, "State(s) in (\"\")"=w921) -> ("States Out"=w920:string)  [unwired: 13 in]
      }
      frame "Control: Read Config" {
        n438 = Unbundle By Name(w934) -> ("last state"=w935:T12)
        n439 = call <userlib>:"Current VIs Parent Directory__ogtk.vi"("Relative path (.)"=path "config.ini") -> ("Parent Directory (+ Relative)"=w949:path)  [unwired: 4 out]
        n440 = call <vilib>:"Open Config Data (compatibility).vi"("error in (no error)"=w940, "configuration file path"=w949) -> ("error out"=w941:errorcluster, "refnum"=w948:T14)  [unwired: 7 in, 1 out]
        n441 = call <userlib>:"Read INI Cluster__ogtk.vi"("error in (no error)"=w941, "INI Fomatted Cluster Type"=w935, "refnum"=w948) -> ("error out"=w942:errorcluster, "INI Fomatted Cluster"=w947:variant, "dup refnum"=w943:T14)  [unwired: 6 out]
        n442 = Variant To Data(error in=w942, type=w935, Variant=w947) -> (data=w936:T12, error out=w928:errorcluster)
        n443 = Bundle By Name(cluster=w934, "last state"=w936) -> (w932:T10)
        n444 = Unbundle By Name(w932) -> ("Control"=w931:refnum<class "Control.lvclass">)
        n445 = call-dynamic "Read Text Font.vi"("error in (no error)"=w928, "Control in"=w931) -> ("error out"=w929:errorcluster, "Font"=w938:T1, "Control out"=w926:refnum<class "Control.lvclass">)  [unwired: 7 out]
        n446 = call <userlib>:"Read INI Cluster__ogtk.vi"("error in (no error)"=w929, "INI Fomatted Cluster Type"=w938, "refnum"=w943) -> ("error out"=w946:errorcluster, "INI Fomatted Cluster"=w944:variant, "dup refnum"=w945:T14)  [unwired: 6 out]
        n447 = Variant To Data(error in=w946, type=w938, Variant=w944) -> (data=w924:T1, error out=w923:errorcluster)
        n448 = call-dynamic "Write Text Font.vi"("error in (no error)"=w923, "Font"=w924, "Control in"=w926) -> ("error out"=w922:errorcluster, "Control out"=w925:refnum<class "Control.lvclass">)  [unwired: 7 out]
        n449 = call <vilib>:"Close Config Data.vi"("error in (no error)"=w922, "refnum"=w945) -> ("error out"=w939:errorcluster)  [unwired: 1 in, 8 out]
        n450 = Bundle By Name(cluster=w932, "Control"=w925) -> (w930:T10)
        n451 = call <vilib>:"Add State(s) to Queue__jki_lib_state_machine.vi"("State(s) in Front (\"\")"="Control: Set to Last State", "State(s) in (\"\")"=w933) -> ("States Out"=w937:string)  [unwired: 13 in]
      }
      frame "Control: Save Config" {
        n452 = Unbundle By Name(w983) -> ("last state"=w966:T12, "Control"=w972:refnum<class "Control.lvclass">)
        n453 = call <userlib>:"Current VIs Parent Directory__ogtk.vi"("Relative path (.)"=path "config.ini") -> ("Parent Directory (+ Relative)"=w989:path)  [unwired: 4 out]
        n454 = call <vilib>:"Open Config Data.vi"("error in (no error)"=w988, "configuration file path"=w989) -> ("error out"=w969:errorcluster, "refnum"=w979:T14)  [unwired: 7 in, 1 out]
        n455 = call-dynamic "Read Action.vi"("error in (no error)"=w969, "Control in"=w972) -> ("error out"=w974:errorcluster, "Action"=w963:T3, "Control out"=w973:refnum<class "Control.lvclass">)  [unwired: 7 out]
        n456 = local read "End program afterwards"() -> (w951:bool)
        n457 = call-dynamic "Read Orientations.vi"("error in (no error)"=w974, "Control in"=w973) -> ("error out"=w977:errorcluster, "Orientations"=w962:T24, "Control out"=w976:refnum<class "Control.lvclass">)  [unwired: 7 out]
        n458 = call-dynamic "Read Style.vi"("error in (no error)"=w977, "Control in"=w976) -> ("error out"=w978:errorcluster, "Style index"=w961:T25, "Control out"=w975:refnum<class "Control.lvclass">)  [unwired: 7 out]
        n459 = call-dynamic "Read Control Text.vi"("error in (no error)"=w978, "Control in"=w975) -> ("error out"=w953:errorcluster, "Control Text"=w960:string, "Control out"=w959:refnum<class "Control.lvclass">)  [unwired: 7 out]
        n460 = local read "Icon source"() -> (w964:path)
        n461 = call-dynamic "Read Text Color.vi"("error in (no error)"=w953, "Control.lvclass in"=w959) -> ("error out"=w952:errorcluster, "Text Color"=w955:u32, "Control.lvclass out"=w958:refnum<class "Control.lvclass">)  [unwired: 7 out]
        n462 = call-dynamic "Read Scale Icon.vi"("error in (no error)"=w952, "Control in"=w958) -> ("error out"=w954:errorcluster, "Scale Icon"=w956:dbl, "Control out"=w957:refnum<class "Control.lvclass">)  [unwired: 7 out]
        n463 = Bundle By Name(cluster=w966, "Scale"=w956, "Text Color"=w955, "Control Text"=w960, "Style"=w961, "Orientations"=w962, "Action"=w963, "Icon png"=w964, "Close afterwards"=w951) -> (w965:T12)
        n464 = call <userlib>:"Write INI Cluster__ogtk.vi"("error in (no error)"=w954, "INI Fomatted Cluster"=w965, "refnum"=w979) -> ("error out"=w968:errorcluster, "dup refnum"=w982:T14)  [unwired: 1 in, 6 out]
        n465 = call-dynamic "Read Text Font.vi"("error in (no error)"=w968, "Control in"=w957) -> ("error out"=w967:errorcluster, "Font"=w970:T1, "Control out"=w971:refnum<class "Control.lvclass">)  [unwired: 7 out]
        n466 = call <userlib>:"Write INI Cluster__ogtk.vi"("error in (no error)"=w967, "INI Fomatted Cluster"=w970, "refnum"=w982) -> ("error out"=w980:errorcluster, "dup refnum"=w981:T14)  [unwired: 1 in, 6 out]
        n467 = Bundle By Name(cluster=w983, "Control"=w971) -> (w984:T10)
        n468 = call <vilib>:"Close Config Data.vi"("error in (no error)"=w980, "refnum"=w981) -> ("error out"=w987:errorcluster)  [unwired: 1 in, 8 out]
        n469 = call <vilib>:"Add State(s) to Queue__jki_lib_state_machine.vi"("State(s) in (\"\")"=w985) -> ("States Out"=w986:string)  [unwired: 14 in]
      }
      frame "Control: Set to Last State" {
        n470 = Unbundle By Name(w1029) -> ("Control"=w1028:refnum<class "Control.lvclass">, "last state"=w1021:T12, "user events"=w1019:T4)
        n471 = call-dynamic "Read Text Font.vi"("error in (no error)"=w1008, "Control in"=w1028) -> ("error out"=w993:errorcluster, "Font"=w1002:T1)  [unwired: 8 out]
        n472 = Unbundle By Name(w1019) -> ("Icon (*.png)"=w1013:refnum<user-event>, "Action"=w1018:refnum<user-event>, "Orientations"=w1016:refnum<user-event>, "Font"=w1004:refnum<user-event>, "Control Text"=w1003:refnum<user-event>, "Style"=w999:refnum<user-event>, "Text Color"=w997:refnum<user-event>, "Scale Icon"=w994:refnum<user-event>)
        n473 = Unbundle By Name(w1021) -> ("Action"=w1017:T3, "Orientations"=w1015:T2, "Icon png"=w1012:path, "Control Text"=w1001:string, "Style"=w998:u16, "Text Color"=w996:u32, "Scale"=w992:dbl, "Close afterwards"=w991:bool)
        n474 = Generate User Event(user event=w994, event data cluster=w992, error in=w993) -> (error out=w995:errorcluster)  [unwired: 1 out]
        n475 = Generate User Event(user event=w997, event data cluster=w996, error in=w995) -> (error out=w1006:errorcluster)  [unwired: 1 out]
        n476 = Generate User Event(user event=w999, event data cluster=w998, error in=w1006) -> (error out=w1000:errorcluster)  [unwired: 1 out]
        n477 = local write "End program afterwards"(w991) -> ()
        n478 = Generate User Event(user event=w1003, event data cluster=w1001, error in=w1000) -> (error out=w1007:errorcluster)  [unwired: 1 out]
        n479 = call-poly <userlib>:"File Exists__ogtk.vi"("file path"=w1012) -> ("exists"=w1027:bool)  [unwired: 6 in, 1 out]
        n480 = Empty String/Path?(string/path=w1012) -> (empty?=w1026:bool)
        n481 = Generate User Event(user event=w1004, event data cluster=w1002, error in=w1007) -> (error out=w1005:errorcluster)  [unwired: 1 out]
        n482 = Generate User Event(user event=w1016, event data cluster=w1015, error in=w1005) -> (error out=w1011:errorcluster)  [unwired: 1 out]
        n483 = Compound Arithmetic op=AND(w1027, invert w1026) -> (w1014:bool)
        n484 = Generate User Event(user event=w1018, event data cluster=w1017, error in=w1011) -> (error out=w1010:errorcluster)  [unwired: 1 out]
        n485 = Select(t="", s=w1014, f="Control: Browse Icon") -> (s? t:f=w1023:string)
        n486 = case shown="True" w1014 {
          tunnel: w1013 -> [_ w1034]
          tunnel: w1012 -> [_ w1033]
          tunnel: w1010 -> [w1030 w1032]
          tunnel: [w1030 w1031] -> w1009
          frame False {
          }
          frame True {
            n487 = Generate User Event(user event=w1034, event data cluster=w1033, error in=w1032) -> (error out=w1031:errorcluster)  [unwired: 1 out]
          }
        }
        n488 = call <vilib>:"Add State(s) to Queue__jki_lib_state_machine.vi"("State(s) in Front (\"\")"=w1023, "State(s) in (\"\")"=w1022) -> ("States Out"=w1020:string)  [unwired: 13 in]
      }
      frame "Control: Browse Icon" {
        n489 = Unbundle By Name(w1041) -> ("Control"=w1042:refnum<class "Control.lvclass">)
        n490 = call <userlib>:"Current VIs Parent Directory__ogtk.vi"("Relative path (.)"=path "config.ini") -> ("Parent Directory (+ Relative)"=w1045:path)  [unwired: 4 out]
        n491 = call "Get Icon Source Path INI.vi"("error in"=w1036, "config.ini path"=w1045) -> ("error out"=w1037:errorcluster, "Icon source dir"=w1044:path, "config.ini path dup"=w1043:path)  [unwired: 1 in, 6 out]
        n492 = call "File Dialog2"("start path"=w1044, "prompt"="Select a single PNG file or choose a source directory for batch processing." ("pattern label"), "error in"=w1037, "pattern (all files)"="*.png", "pattern label"="PNG files") -> ("selected path"=w1047:path, "cancelled"=w1050:bool, "error out"=w1051:errorcluster)  [unwired: 2 in, 6 out]
        n493 = case shown="False" w1050 {
          tunnel: [w1067 w1072] -> w1039
          tunnel: w1042 -> [w1065 w1072]
          tunnel: w1051 -> [w1064 w1070]
          tunnel: [w1062 w1069] -> w1035
          tunnel: w1047 -> [w1061 _]
          tunnel: w1043 -> [w1057 _]
          tunnel: ["Preview" ("State(s) in Front (\"\")") "Error >> 7001" ("State(s) in Front (\"\")")] -> w1038
          frame False {
            n494 = local write "Icon source"(w1061) -> ()
            n495 = call-poly <userlib>:"Strip Path__ogtk.vi"("path"=w1061) -> ("stripped path"=w1056:path, "name"=w1060:string)
            n496 = call-poly <userlib>:"Strip Path Extension__ogtk.vi"("path"=w1060) -> ("root"=w1059:string)  [unwired: 1 out]
            n497 = call-dynamic "Load Icon.vi"("error in (no error)"=w1064, "Icon path False"=w1061, "Control in"=w1065) -> ("error out"=w1063:errorcluster, "Control out"=w1066:refnum<class "Control.lvclass">)  [unwired: 1 in, 6 out]
            n498 = call-poly <userlib>:"To Proper Case__ogtk.vi"("string"=w1059) -> ("proper case string"=w1058:string)  [unwired: 4 out]
            n499 = local write "Control Text"(w1058) -> ()
            n500 = call "Set Icon Source Path INI.vi"("Icon source dir"=w1056, "config.ini path"=w1057) -> ()  [unwired: 1 in, 9 out]
            n501 = call-dynamic "Write Control Text.vi"("error in (no error)"=w1063, "Control Text"=w1058, "Control in"=w1066) -> ("error out"=w1062:errorcluster, "Control out"=w1067:refnum<class "Control.lvclass">)  [unwired: 7 out]
          }
          frame True {
            n502 = Unbundle By Name(w1070) -> ("code"=w1071:i32)
            n503 = case shown="Default" w1071 {
              tunnel: [w1073 w1074] -> w1069
              tunnel: w1070 -> [w1073 w1075]
              frame Default {
              }
              frame 43 {
                n504 = call <vilib>:"Clear Errors.vi"("error in (no error)"=w1075) -> ("error out"=w1074:errorcluster)  [unwired: 6 out]
              }
            }
          }
        }
        n505 = Bundle By Name(cluster=w1041, "Control"=w1039) -> (w1040:T10)
        n506 = call <vilib>:"Add State(s) to Queue__jki_lib_state_machine.vi"("State(s) in Front (\"\")"=w1038, "State(s) in (\"\")"=w1054) -> ("States Out"=w1053:string)  [unwired: 13 in]
      }
    }
  }
